vi "calibration_main.vi"() -> ()   [LabVIEW 2019]
uses:
  <vilib>/vision/Calibration.llb/Error Statistics.ctl
  LinearTransformationDescriptionCluster.ctl
  <vilib>/vision/driver/IMAQdx.llb/IMAQdx Acquisition Mode.ctl
  <vilib>/vision/Calibration.llb/Distortion Model.ctl
  <vilib>/vision/Calibration.llb/Distortion Model Types.ctl
  CalibrationStepsEnum.ctl
  CircleDetectionEnum.ctl
  <vilib>/vision/Calibration.llb/Calibration Reference Points.ctl
  radiucenter2topleftwidthheight.vi
  affine_transform_point.vi
  ParametersGlobal.vi
  <vilib>/vision/driver/NI_Vision_Acquisition_Software.lvlib
  <vilib>/vision/NI_Vision_Development_Module.lvlib
panel:
  in  "Camera":bool
  in  "Configure Projector and Calibrate Power for Tag:\n(Blank if N/A, nonblank skips Spatial Calibration)":string
  out "error out":errorcluster
  out "Parameters Written":string[][](array[string])
  in  "Power Meter Probe Area (mm^2)":dbl=71.0 format="%#_13g"
  in  "Power":bool
  out "Error Map":sgl[][](graph)
  out "distortion corrected std":dbl format="%0.2f"
  out "linear std":dbl format="%0.2f"
  out "distortion corrected error mean (camera pixels)":dbl format="%0.2f"
  out "linear mean error (camera pixels)":dbl format="%0.2f"
  out "Calibration Instructions":string="Calibration Has Not Started"
  in  "Next Step":bool
  out "Linear Tranformation Description":T1 {"mean error\n(projector pixels)" format="%0.2f"}
  out "Projector  to Camera\nError Statistics (pixels)":T2
  out "grid step (camera pixels)":dbl
  out "mean linear error\n(projector pixels)":dbl format="%0.2f"
  out "Stimulus Image":T3(plugin-control)
  out "ProjectorXY":cluster{"X":dbl, "Y":dbl}[](graph)
  out "CameraXY":cluster{"X":dbl, "Y":dbl}[](graph)
  out "CorrectionMetric":dbl
  out "Spiral Iteration":i32
  in  "ProjectedRadiusFactor":dbl=0.1 format="%#_13g"
  out "CameraToProjectorCorrection":dbl
  out "Circles Data":T4(array[cluster])
  out "Real World\nError Statistics (mm)":T5
  out "Processed Image":T3(plugin-control)
  out "Acquired Image":T3(plugin-control)
  # "Skip Calibration If Possible For:"
  # "Things you need before starting:\n(?) An agar plate with calibration grid paper with\n     0.25mm spacing (1/4 size). This is only required \n     if camera needs to be calibrated\n(?) An agar plate with plain paper\n(-) An agar plate with no paper\n(?) A power meter on an a 9cm plate (no agar)\n     This is only required for power calibration"
  # "If this % distortion is > 1%\nSomething is probably wrong"
  # "±"
  # "±"
  # "C:/Users/Public/Documents/National Instruments/Vision/Documentation/CalibrationGrid.pdf"
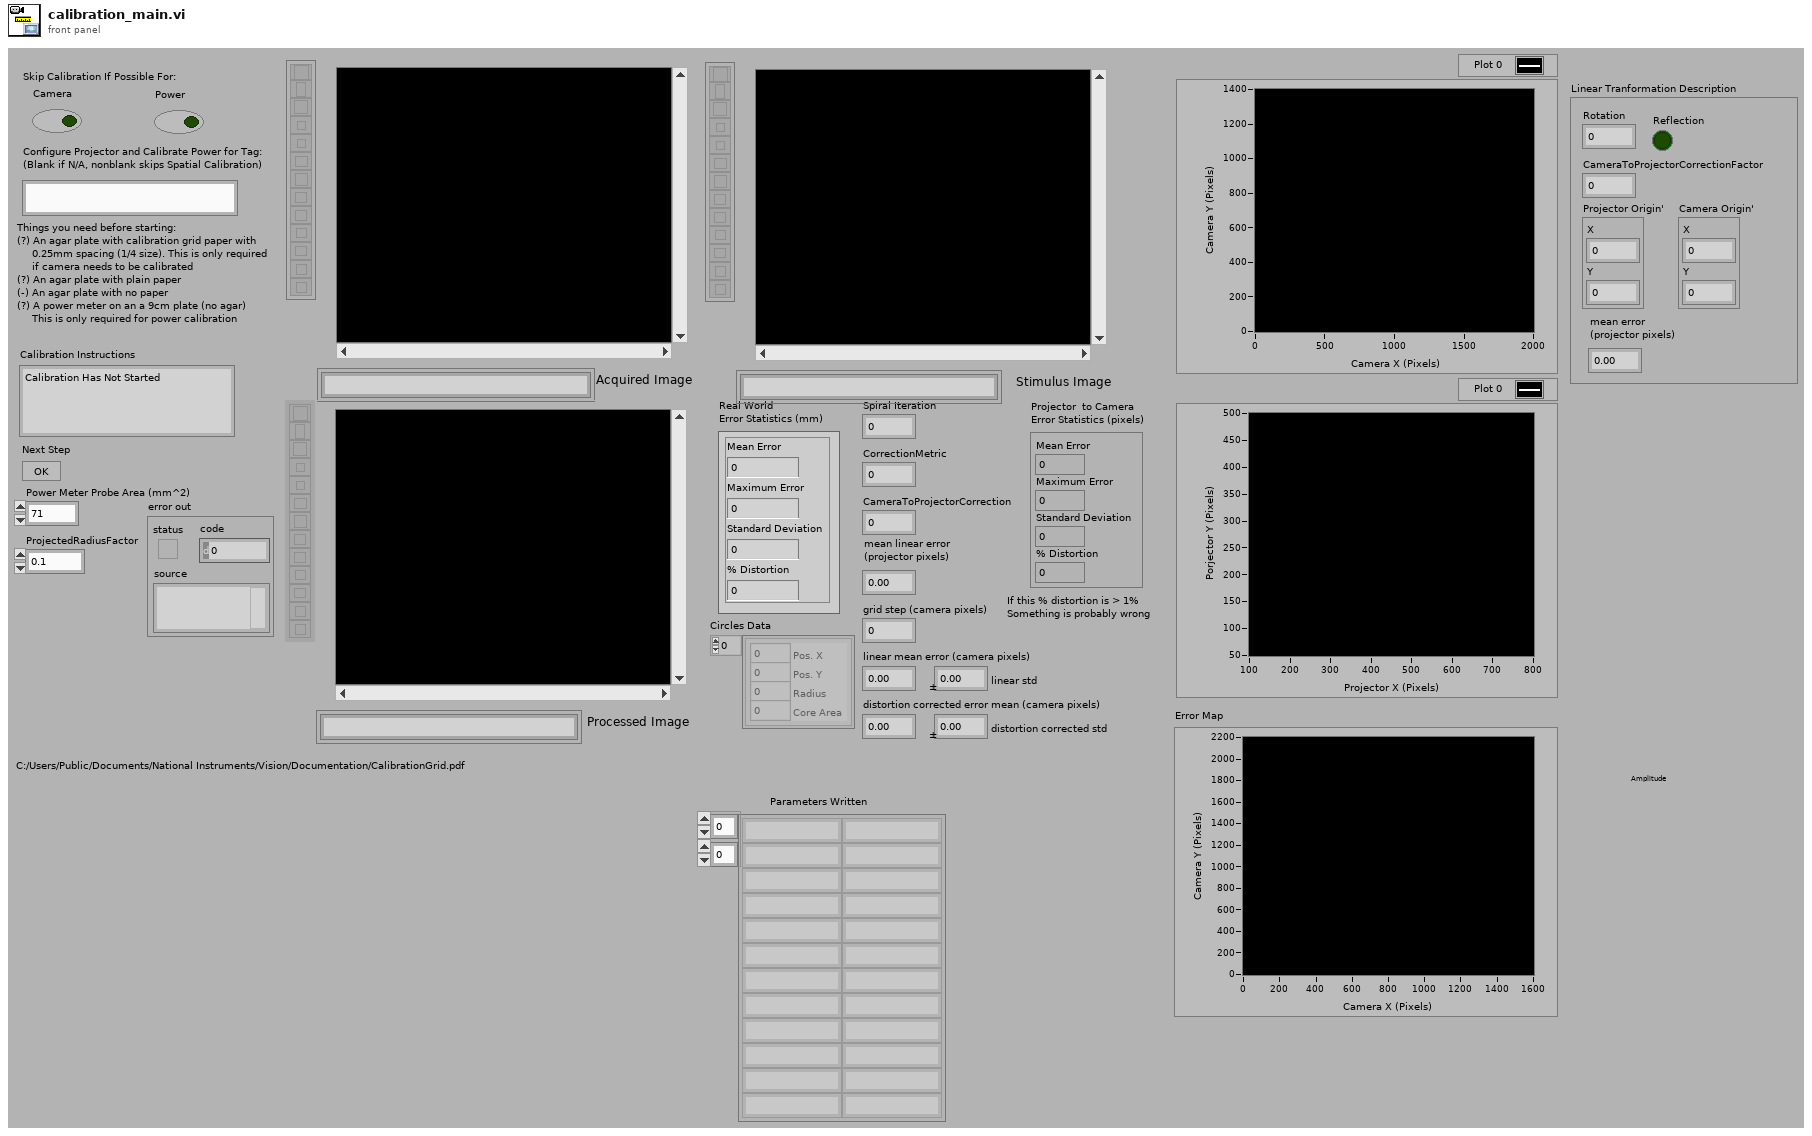
[diagram p1: front panel]
types:
  T1 = typedef "LinearTransformationDescriptionCluster.ctl" = cluster{"Rotation":sgl, "Reflection":bool, "CameraToProjectorCorrectionFactor":dbl, "Projector Origin'":cluster{"X":dbl, "Y":dbl}, "Camera Origin'":cluster{"X":dbl, "Y":dbl}, "mean error\n(projector pixels)":dbl}
  T2 = typedef "Error Statistics.ctl" = cluster{"Mean Error":dbl, "Maximum Error":dbl, "Standard Deviation":dbl, "% Distortion":dbl}
  T3 = typedef "IMAQ Image.ctl" = refnum<image>
  T4 = cluster{"Pos. X":i32, "Pos. Y":i32, "Radius":i32, "Core Area":i32}[]
  T5 = cluster{"Mean Error":dbl, "Maximum Error":dbl, "Standard Deviation":dbl, "% Distortion":dbl}
  T6 = typedef "NI_Vision_Acquisition_Software.lvlib/IMAQdx Acquisition Mode.ctl" = enum32{"One Shot", "Continuous"}
  T7 = typedef "Image Type" = u32
  T8 = typedef "IMAQdx.ctl" = refnum<k21>
  T9 = typedef "Image Unit" = enum32{"Undefined", "Angström", "Micrometer", "Millimeter", "Centimeter", "Meter", "Kilometer", "Microinch", "Inch", "Feet", "Nautical miles", "Standard miles", "Steps"}
  T10 = typedef "CalibrationStepsEnum.ctl" = enum16{"FindSpot", "SpiralScan", "CalculatingLinearTranformation", "CalculatingNonlinearTransformation", "CalibrationError", "CalibrationComplete"}
  T11 = typedef "CircleDetectionEnum.ctl" = enum16{"NoCircle", "CircleCutoff", "CircleFull"}
  T12 = enum32{"AutoM", "Close", "Dilate", "Erode", "Gradient", "Gradient in", "Gradient out", "HitMiss", "Open", "PClose", "POpen", "Thick", "Thin"}
  T13 = typedef "Calibration Reference Points.ctl" = cluster{"Pixel Coordinates":cluster{"X":dbl, "Y":dbl}[], "Real World Coordinates":cluster{"X":dbl, "Y":dbl}[], "Unit":T9, "Image Size":cluster{"X":u32, "Y":u32}}
  T14 = typedef "Distortion Model.ctl" = cluster{"Distortion Model":T15, "Polynomial Model Setup":cluster{"Radial Coefficient":u32, "Tangential Coefficients ":bool}}
  T15 = typedef "Distortion Model Types.ctl" = i32
  T16 = typedef "Particle Parameters" = i32
  T17 = cluster{"Measurement Parameter":T16, "Range Lower Value":dbl, "Range Upper Value":dbl, "Range":bool, "Measurement Type":bool}[]
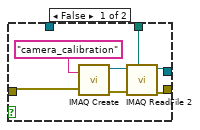
[diagram p3: hidden frame]
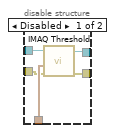
[diagram p5: hidden frame]
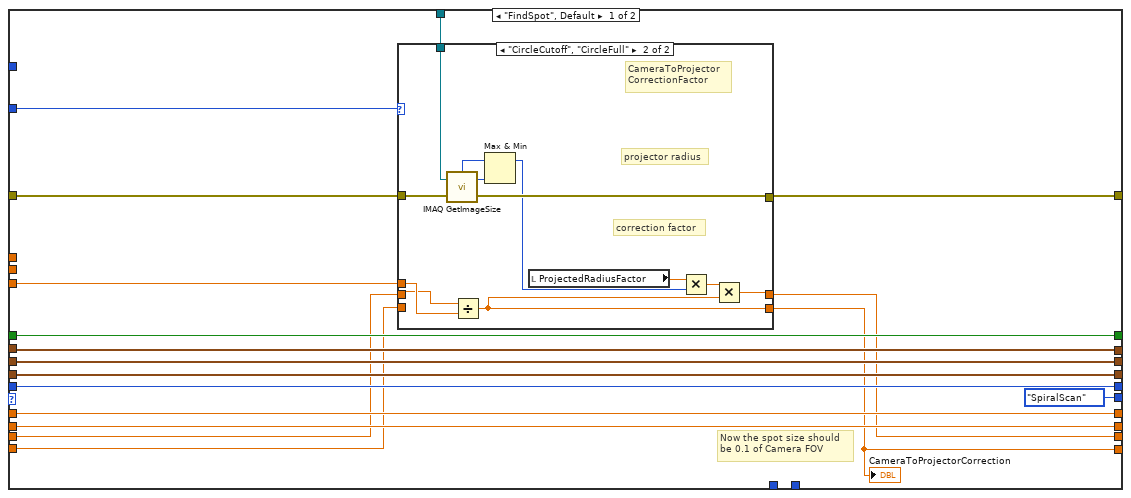
[diagram p7: hidden frame]
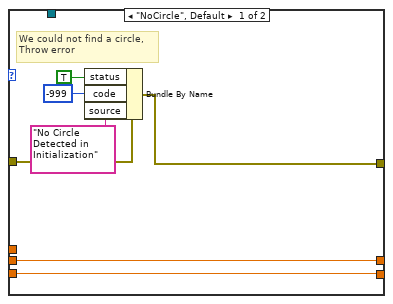
[diagram p8: hidden frame]
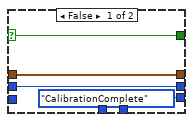
[diagram p11: hidden frame]
diagram:
  # "parameter, value pairs to update parameters.csv"
  # "computer name"
  n1 = String To IP(1:"") -> (0:w38:u32)
  n2 = IP To String(1:FALSE, 2:w38) -> (0:w37:string)
  n3 = Match Pattern(string=w37, regular expression="\\.") -> (before substring=w29:string)  [unwired: 1 in, 3 out]
  n4 = Initialize Array("", 0 ("dimension size"), 2 ("dimension size")) -> (w26:string[][])
  n5 = Not Equal?(x="Configure Projector and Calibrate Power for Tag:\n(Blank if N/A, nonblank skips Spatial Calibration)", y="") -> (x != y?=w28:bool)
  n6 = case shown="True" w28 {
    tunnel: w29 -> [w39 w43]
    tunnel: [w39 w42] -> w23
    tunnel: "Configure Projector and Calibrate Power for Tag:\n(Blank if N/A, nonblank skips Spatial Calibration)" -> [_ w45]
    frame False {
    }
    frame True {
      w41 = ";" ("delimiter")
      n7 = call <vilib>:"Space Constant.vi"() -> ("String"=w46:string)
      n8 = call <vilib>:"Delimited String to 1D String Array.vi"("delimiter"=w46, "delimited string"=w45) -> ("string array"=w44:string[])  [unwired: 9 in]
      n9 = call <vilib>:"1D String Array to Delimited String.vi"("delimiter"=w41, "string array"=w44) -> ("delimited string"=w40:string)  [unwired: 9 in]
      n10 = Concatenate Strings(w43, w41, w40) -> (w42:string)
    }
  }
  n11 = flat-sequence {
    tunnel: "Configure Projector and Calibrate Power for Tag:\n(Blank if N/A, nonblank skips Spatial Calibration)" -> [w49]
    tunnel: w26 -> [w54]
    tunnel: w23 -> [w53]
    tunnel: [w49] -> w22
    tunnel: [w54] -> w21
    tunnel: [w53] -> w20
    tunnel: [w48] -> w5
    tunnel: [w47] -> w2
    tunnel: [w110] -> w24
    tunnel: [w111] -> w25
    tunnel: w22 -> [w63]
    tunnel: w21 -> [w111]
    tunnel: w20 -> [w110]
    tunnel: [w75] -> w19
    tunnel: [w74] -> w18
    tunnel: [w66] -> w17
    tunnel: [w65] -> w16
    tunnel: [w62] -> w6
    tunnel: w2 -> [w60]
    tunnel: [w56] -> w1
    frame #0 {
      # "allow resolution mismatch"
      n12 = call "load_parameters.vi"("Create Data Folder (T)"=FALSE, "Tags"=w49) -> ("error out"=w52:errorcluster, "Computer Found"=w48:bool)  [unwired: 7 in, 1 out]
      n13 = call <vilib>:"Clear Errors.vi"("error in (no error)"=w52, "specific error code to clear (0: all)"=-919) -> ("error out"=w47:errorcluster)  [unwired: 4 in, 1 out]
      n14 = local write "Calibration Instructions"("Starting Calibration... Please Wait") -> ()
    }
    frame #1 {
      w68 = u32 20  # Number of Buffers
      w67 = IMAQdx_Acquisition_Mode."Continuous"  # Continuous?
      w81 = T7 4 items=["Grayscale (U8)", "Grayscale (I16)", "Grayscale (SGL)", "Complex (CSG)", "RGB (U32)", "HSL (U32)", "RGB (U64)"] ("Image Type")
      w77 = T7 4 items=["Grayscale (U8)", "Grayscale (I16)", "Grayscale (SGL)", "Complex (CSG)", "RGB (U32)", "HSL (U32)", "RGB (U64)"] ("Image Type")
      # "The stimulus Image has half the verticle resolution for 4500s"
      # "display full field image"
      n15 = global read "ParametersGlobal.vi" "Projector Calibration Points"() -> (w106:cluster{"X":dbl, "Y":dbl}[])
      n16 = global read "ParametersGlobal.vi" "PureGreenExposureTime"() -> (w58:i32)
      n17 = Array Size(array=w106) -> (size(s)=w107:i32)
      n18 = call "initialize_projector.vi"("Green Only"=TRUE, "error in"=w60, "green exp_time_us"=w58) -> ("error out"=w59:errorcluster)  [unwired: 8 in]
      n19 = Equal To 0?(x=w107) -> (x = 0?=w108:bool)
      n20 = Not Equal?(x=w63, y="") -> (x != y?=w62:bool)
      n21 = And(x=w108, y=w62) -> (x .and. y?=w109:bool)
      n22 = case shown="True" w109 {
        tunnel: [w115 w116] -> w64
        tunnel: w59 -> [w115 w119]
        frame False {
        }
        frame True {
          # "require tags to have previous calibration"
          n23 = call <vilib>:"Simple Error Handler.vi"("error code (no error:0)"=-723, "error source (\" \")"="Attepting to calibrate for a tag without a previous spatial calibration" ("error source (\" \")"), "error in (no error)"=w119) -> ("error out"=w116:errorcluster)  [unwired: 2 in, 4 out]
        }
      }
      n24 = call "setup_window_display.vi"("error in (no error)"=w64) -> ("error out"=w103:errorcluster, "Height"=w105:i16, "Width"=w104:i16)  [unwired: 8 in]
      n25 = case shown="Error .." w64 {
        selector: w64 -> [_ w112]
        frame No Error {
        }
        frame Error {
          n26 = flat-sequence {
            tunnel: w112 -> [w113]
            frame #0 {
              n27 = local write "error out"(w113) -> ()
            }
            frame #1 {
              n28 = Stop(stop? (T)=TRUE) -> ()
            }
          }
        }
      }
      n29 = call "IMAQ WindZoom 2"("error in (no error)"=w103, "Zoom to Fit? (False)"=TRUE ("Zoom to Fit? (T)")) -> ("error out"=w91:errorcluster)  [unwired: 6 in, 3 out]
      n30 = call "IMAQ Create"("Border Size"=0, "Image Name"="StimulusImage", "Image Type"=w81) -> ("New Image"=w92:T3, "error out"=w96:errorcluster)  [unwired: 2 in]
      n31 = call "IMAQ Create"("Border Size"=0, "Image Name"="DisplayImage", "Image Type"=w77, "error in (no error)"=w91) -> ("New Image"=w90:T3, "error out"=w89:errorcluster)  [unwired: 1 in]
      n32 = call "IMAQ SetImageSize"("error in (no error)"=w89, "Y Resolution"=w105, "X Resolution"=w104, "Image"=w90) -> ("error out"=w102:errorcluster, "Image Out"=w99:T3)  [unwired: 1 in]
      n33 = Divide(x=w105, y=2) -> (x/y=w95:dbl)
      n34 = Round Toward -Infinity(1:w95) -> (0:w94:dbl)
      n35 = global read "ParametersGlobal.vi" "IMAQdx Session"() -> (w69:T8)
      n36 = call "IMAQ SetImageSize"("error in (no error)"=w96, "Y Resolution"=w94, "X Resolution"=w104, "Image"=w92) -> ("error out"=w97:errorcluster, "Image Out"=w93:T3)  [unwired: 1 in]
      n37 = call "IMAQ FillImage"("Color Pixel Value"=u32 0, "error in (no error)"=w97, "Image"=w93) -> ("error out"=w98:errorcluster, "Image Out"=w56:T3)  [unwired: 7 in]
      n38 = local write "Next Step"(FALSE) -> ()
      n39 = call "IMAQ Expand"("Y Duplication Step"=2, "error in (no error)"=w98, "Image Dst"=w99, "Image Src"=w56) -> ("error out"=w101:errorcluster, "Image Dst Out"=w57:T3)  [unwired: 6 in]
      n40 = call <vilib>:"IMAQdx Open Camera.vi"("Session In"=w69) -> ("error out"=w72:errorcluster, "Session Out"=w73:T8)  [unwired: 9 in]
      n41 = Merge Errors(w101, w102) -> (w100:errorcluster)
      n42 = call "IMAQ WindDraw"("Resize to Image Size? (Y)"=FALSE, "error in (no error)"=w100, "Image"=w57) -> ("error out"=w75:errorcluster, "Image Out (duplicate)"=w74:T3)  [unwired: 7 in]
      n43 = call <vilib>:"IMAQdx Configure Acquisition.vi"("error in"=w72, "Number of Buffers"=w68, "Continuous?"=w67, "Session In"=w73) -> ("error out"=w71:errorcluster, "Session Out"=w70:T8)  [unwired: 6 in]
      n44 = call <vilib>:"IMAQdx Start Acquisition.vi"("error in"=w71, "Session In"=w70) -> ("error out"=w66:errorcluster, "Session Out"=w65:T8)  [unwired: 8 in]
    }
  }
  n45 = Not(x=w6) -> (.not. x?=w3:bool)
  n46 = And(x=w3, y=w5) -> (x .and. y?=w4:bool)
  n47 = case shown="True" w3 {
    tunnel: w25 -> [w126 w140]
    tunnel: w24 -> [w125 w139]
    tunnel: w1 -> [w122 w138]
    tunnel: w19 -> [w120 w137]
    tunnel: w18 -> [w121 w136]
    tunnel: w17 -> [w123 w135]
    tunnel: w16 -> [w124 w134]
    tunnel: [w125 w133] -> w13
    tunnel: [w124 w132] -> w12
    tunnel: [w122 w131] -> w11
    tunnel: [w121 w130] -> w10
    tunnel: [w120 w129] -> w9
    tunnel: [w126 w128] -> w8
    tunnel: [w123 w127] -> w7
    frame False {
    }
    frame True {
      # "do spatial calibration"
      n48 = flat-sequence {
        tunnel: [w310] -> w308
        tunnel: [w326] -> w307
        tunnel: [w325] -> w306
        tunnel: [w324] -> w305
        tunnel: [w312] -> w304
        tunnel: [w311] -> w303
        tunnel: [w323] -> w302
        tunnel: [w313] -> w301
        tunnel: [w322] -> w300
        tunnel: w134 -> [w324]
        tunnel: w135 -> [w310]
        tunnel: w136 -> [w326]
        tunnel: w137 -> [w325]
        tunnel: w138 -> [w323]
        tunnel: w140 -> [w322]
        tunnel: w139 -> [w313]
        tunnel: w308 -> [w362]
        tunnel: [w358] -> w294
        tunnel: [w383] -> w295
        tunnel: [w382] -> w296
        tunnel: w307 -> [w383]
        tunnel: w306 -> [w382]
        tunnel: w305 -> [w358]
        tunnel: w304 -> [w363]
        tunnel: w303 -> [w360]
        tunnel: [w335] -> w297
        tunnel: [w334] -> w298
        tunnel: w302 -> [w356]
        tunnel: [w356] -> w299
        tunnel: w301 -> [w343]
        tunnel: [w343] -> w293
        tunnel: w300 -> [w342]
        tunnel: [w338] -> w292
        tunnel: w299 -> [w400]
        tunnel: [w399] -> w284
        tunnel: w298 -> [w412]
        tunnel: [w412] -> w285
        tunnel: w297 -> [w411]
        tunnel: [w411] -> w286
        tunnel: w296 -> [w395]
        tunnel: [w397] -> w287
        tunnel: w295 -> [w396]
        tunnel: [w398] -> w288
        tunnel: w294 -> [w410]
        tunnel: [w410] -> w289
        tunnel: w293 -> [w408]
        tunnel: [w408] -> w290
        tunnel: w292 -> [w407]
        tunnel: [w407] -> w291
        tunnel: [w423] -> w283
        tunnel: [w422] -> w282
        tunnel: [w421] -> w281
        tunnel: [w420] -> w280
        tunnel: [w419] -> w279
        tunnel: w291 -> [w419]
        tunnel: w290 -> [w420]
        tunnel: w289 -> [w421]
        tunnel: w288 -> [w417]
        tunnel: w287 -> [w416]
        tunnel: w286 -> [w422]
        tunnel: w285 -> [w423]
        tunnel: w284 -> [w415]
        tunnel: [w417] -> w278
        tunnel: [w416] -> w277
        tunnel: [w415] -> w276
        tunnel: w283 -> [w438]
        tunnel: [w438] -> w275
        tunnel: w282 -> [w430]
        tunnel: [w428] -> w274
        tunnel: [w425] -> w273
        tunnel: [w426] -> w272
        tunnel: w281 -> [w429]
        tunnel: [w429] -> w271
        tunnel: w280 -> [w437]
        tunnel: [w437] -> w270
        tunnel: w279 -> [w436]
        tunnel: [w436] -> w269
        tunnel: [w427] -> w268
        tunnel: w278 -> [w426]
        tunnel: w277 -> [w425]
        tunnel: [w424] -> w267
        tunnel: w276 -> [w424]
        tunnel: [w440] -> w266
        tunnel: w275 -> [w456]
        tunnel: [w456] -> w265
        tunnel: w274 -> [w455]
        tunnel: [w455] -> w264
        tunnel: w273 -> [w443]
        tunnel: [w442] -> w263
        tunnel: w272 -> [w444]
        tunnel: [w441] -> w262
        tunnel: w271 -> [w454]
        tunnel: [w454] -> w261
        tunnel: w270 -> [w453]
        tunnel: [w453] -> w260
        tunnel: w269 -> [w452]
        tunnel: [w452] -> w259
        tunnel: w268 -> [w451]
        tunnel: [w451] -> w258
        tunnel: w267 -> [w439]
        tunnel: w266 -> [w473]
        tunnel: [w473] -> w257
        tunnel: w265 -> [w472]
        tunnel: [w472] -> w256
        tunnel: w264 -> [w469]
        tunnel: [w462] -> w255
        tunnel: w263 -> [w471]
        tunnel: [w471] -> w254
        tunnel: w262 -> [w470]
        tunnel: [w470] -> w253
        tunnel: w261 -> [w468]
        tunnel: [w468] -> w252
        tunnel: [w461] -> w251
        tunnel: [w460] -> w250
        tunnel: w260 -> [w460]
        tunnel: w259 -> [w459]
        tunnel: [w459] -> w249
        tunnel: [w458] -> w248
        tunnel: w258 -> [w458]
        tunnel: [w509] -> w247
        tunnel: [w508] -> w246
        tunnel: [w505] -> w245
        tunnel: w257 -> [w500]
        tunnel: w256 -> [w481]
        tunnel: w255 -> [w506]
        tunnel: w254 -> [w502]
        tunnel: w253 -> [w507]
        tunnel: w252 -> [w504]
        tunnel: [w504] -> w244
        tunnel: [w485] -> w243
        tunnel: [w484] -> w242
        tunnel: [w482] -> w241
        tunnel: [w481] -> w240
        tunnel: w251 -> [w480]
        tunnel: [w480] -> w239
        tunnel: w250 -> [w476]
        tunnel: [w476] -> w238
        tunnel: w249 -> [w475]
        tunnel: [w475] -> w237
        tunnel: w248 -> [w474]
        tunnel: w247 -> [w913]
        tunnel: [w913] -> w236
        tunnel: w246 -> [w909]
        tunnel: [w909] -> w235
        tunnel: w245 -> [w908]
        tunnel: [w907] -> w234
        tunnel: w244 -> [w912]
        tunnel: [w912] -> w233
        tunnel: w243 -> [w911]
        tunnel: w242 -> [w910]
        tunnel: [w903] -> w232
        tunnel: w241 -> [w906]
        tunnel: [w906] -> w231
        tunnel: w240 -> [w905]
        tunnel: [w905] -> w230
        tunnel: w239 -> [w904]
        tunnel: [w904] -> w229
        tunnel: [w903] -> w228
        tunnel: w238 -> [w902]
        tunnel: [w902] -> w227
        tunnel: w237 -> [w901]
        tunnel: [w901] -> w226
        tunnel: w236 -> [w960]
        tunnel: [w961] -> w225
        tunnel: w235 -> [w967]
        tunnel: [w931] -> w224
        tunnel: w234 -> [w971]
        tunnel: [w959] -> w223
        tunnel: w233 -> [w972]
        tunnel: [w972] -> w222
        tunnel: w232 -> [w956]
        tunnel: w231 -> [w968]
        tunnel: w230 -> [w958]
        tunnel: [w937] -> w221
        tunnel: [w915] -> w220
        tunnel: [w958] -> w219
        tunnel: [w916] -> w218
        tunnel: [w922] -> w217
        tunnel: w229 -> [w957]
        tunnel: [w957] -> w216
        tunnel: [w946] -> w215
        tunnel: w228 -> [w941]
        tunnel: [w941] -> w214
        tunnel: w227 -> [w933]
        tunnel: [w933] -> w213
        tunnel: w226 -> [w918]
        tunnel: [w928] -> w212
        tunnel: w225 -> [w1074]
        tunnel: [w1074] -> w211
        tunnel: w224 -> [w1073]
        tunnel: [w1073] -> w210
        tunnel: w223 -> [w1072]
        tunnel: [w1009] -> w209
        tunnel: w222 -> [w1071]
        tunnel: [w1071] -> w208
        tunnel: w221 -> [w1063]
        tunnel: w220 -> [w1062]
        tunnel: w219 -> [_]
        tunnel: w218 -> [_]
        tunnel: w217 -> [w1059]
        tunnel: w216 -> [w1067]
        tunnel: [w1067] -> w207
        tunnel: w215 -> [w992]
        tunnel: [w1052] -> w206
        tunnel: [w993] -> w205
        tunnel: w214 -> [w1065]
        tunnel: [w1065] -> w204
        tunnel: w213 -> [w1061]
        tunnel: [w1061] -> w203
        tunnel: w212 -> [w995]
        tunnel: [w1022] -> w202
        tunnel: [w1008] -> w201
        tunnel: [w1059] -> w200
        tunnel: [w1053] -> w199
        tunnel: [w1031] -> w198
        tunnel: [w992] -> w197
        tunnel: w211 -> [w1085]
        tunnel: w210 -> [w1084]
        tunnel: w209 -> [w1097]
        tunnel: [w1096] -> w186
        tunnel: w208 -> [w1102]
        tunnel: [w1102] -> w187
        tunnel: w207 -> [w1101]
        tunnel: [w1101] -> w188
        tunnel: w206 -> [w1098]
        tunnel: w205 -> [w1094]
        tunnel: w204 -> [w1099]
        tunnel: w203 -> [w1089]
        tunnel: [w1089] -> w189
        tunnel: w202 -> [w1088]
        tunnel: [w1088] -> w190
        tunnel: [w1081] -> w191
        tunnel: w201 -> [w1081]
        tunnel: w200 -> [w1086]
        tunnel: [w1086] -> w192
        tunnel: [w1085] -> w193
        tunnel: [w1084] -> w194
        tunnel: w199 -> [w1083]
        tunnel: [w1083] -> w195
        tunnel: w198 -> [w1082]
        tunnel: [w1082] -> w196
        tunnel: [w1080] -> w185
        tunnel: w197 -> [w1080]
        tunnel: [w1117] -> w184
        tunnel: [w1124] -> w183
        tunnel: [w1127] -> w182
        tunnel: [w1126] -> w181
        tunnel: [w1122] -> w180
        tunnel: [w1120] -> w179
        tunnel: [w1121] -> w178
        tunnel: [w1125] -> w177
        tunnel: [w1123] -> w176
        tunnel: [w1119] -> w175
        tunnel: [w1112] -> w174
        tunnel: [w1111] -> w173
        tunnel: w196 -> [w1119]
        tunnel: w195 -> [w1123]
        tunnel: w194 -> [w1125]
        tunnel: w193 -> [w1121]
        tunnel: w192 -> [w1120]
        tunnel: w191 -> [w1122]
        tunnel: w190 -> [w1126]
        tunnel: w189 -> [w1127]
        tunnel: w188 -> [w1124]
        tunnel: w187 -> [w1117]
        tunnel: w186 -> [w1118]
        tunnel: [w1108] -> w172
        tunnel: w185 -> [w1108]
        tunnel: [w1137] -> w171
        tunnel: [w1136] -> w170
        tunnel: w184 -> [w1149]
        tunnel: [w1149] -> w169
        tunnel: w183 -> [w1148]
        tunnel: [w1148] -> w168
        tunnel: w182 -> [w1147]
        tunnel: [w1147] -> w167
        tunnel: w181 -> [w1146]
        tunnel: [w1146] -> w166
        tunnel: w180 -> [w1145]
        tunnel: [w1145] -> w165
        tunnel: [w1138] -> w164
        tunnel: w179 -> [w1135]
        tunnel: w178 -> [w1134]
        tunnel: w177 -> [w1133]
        tunnel: w176 -> [w1132]
        tunnel: w175 -> [w1131]
        tunnel: [w1132] -> w163
        tunnel: [w1131] -> w162
        tunnel: w174 -> [w1130]
        tunnel: [w1130] -> w161
        tunnel: w173 -> [w1129]
        tunnel: [w1129] -> w160
        tunnel: [w1128] -> w159
        tunnel: w172 -> [w1128]
        tunnel: [w1173] -> w158
        tunnel: [w1185] -> w157
        tunnel: [w1160] -> w156
        tunnel: [w1184] -> w155
        tunnel: [w1180] -> w154
        tunnel: [w1178] -> w153
        tunnel: [w1170] -> w152
        tunnel: w171 -> [w1173]
        tunnel: w170 -> [w1185]
        tunnel: w169 -> [w1184]
        tunnel: w168 -> [w1174]
        tunnel: w167 -> [w1180]
        tunnel: w166 -> [w1179]
        tunnel: w165 -> [w1165]
        tunnel: w164 -> [w1170]
        tunnel: w163 -> [_]
        tunnel: w162 -> [w1171]
        tunnel: w161 -> [w1167]
        tunnel: w160 -> [w1155]
        tunnel: w159 -> [w1154]
        tunnel: [w1154] -> w151
        tunnel: [w1153] -> w150
        tunnel: w158 -> [w1197]
        tunnel: [w1197] -> w141
        tunnel: w157 -> [w1196]
        tunnel: [w1196] -> w142
        tunnel: w156 -> [w1195]
        tunnel: [w1195] -> w143
        tunnel: w155 -> [w1194]
        tunnel: [w1194] -> w144
        tunnel: w154 -> [w1193]
        tunnel: [w1193] -> w145
        tunnel: w153 -> [w1192]
        tunnel: [w1192] -> w146
        tunnel: w152 -> [w1191]
        tunnel: [w1191] -> w147
        tunnel: w151 -> [w1190]
        tunnel: [w1190] -> w148
        tunnel: w150 -> [w1189]
        tunnel: [w1189] -> w149
        tunnel: [w1212] -> w133
        tunnel: [w1211] -> w132
        tunnel: [w1206] -> w131
        tunnel: [w1207] -> w130
        tunnel: [w1208] -> w129
        tunnel: [w1210] -> w128
        tunnel: [w1209] -> w127
        tunnel: w149 -> [w1204]
        tunnel: w148 -> [w1205]
        tunnel: w147 -> [w1206]
        tunnel: w146 -> [w1210]
        tunnel: w145 -> [w1212]
        tunnel: w144 -> [w1211]
        tunnel: w143 -> [w1203]
        tunnel: w142 -> [w1208]
        tunnel: w141 -> [w1207]
        frame #0 {
          n49 = Concatenate Strings("..\\", w313, "_camera_calibration.png") -> (w316:string)
          n50 = Current VI's Path() -> (path=w320:path)
          n51 = Build Path(base path=w320, name or relative path=w316) -> (appended path=w311:path)
          n52 = call <vilib>:"Check if File or Folder Exists.vi"("path"=w311) -> ("file or folder exists?"=w319:bool)  [unwired: 8 in, 2 out]
          n53 = Not(x="Camera") -> (.not. x?=w314:bool)
          n54 = Not(x=w319) -> (.not. x?=w318:bool)
          n55 = Or(x=w318, y=w314) -> (x .or. y?=w312:bool)
          n56 = local write "Calibration Instructions"("Load dot calibration plate. Turn on IR") -> ()
          n57 = while {
            tunnel: w312 -> [w328]
            stop <- w330 stop-if-true
            n58 = local read "Next Step"() -> (w329:bool)
            n59 = Not(x=w328) -> (.not. x?=w327:bool)
            n60 = Wait (ms)(milliseconds to wait=500) -> ()  [unwired: 1 out]
            n61 = Or(x=w327, y=w329) -> (x .or. y?=w330:bool)
          }
        }
        frame #1 {
          w373 = T14 {"Distortion Model"=0, "Polynomial Model Setup"={"Radial Coefficient"=1, "Tangential Coefficients "=TRUE}}  # Distortion Model Setup
          w374 = T17 [{"Measurement Parameter"=35, "Range Lower Value"=0.0, "Range Upper Value"=1000.0, "Range"=FALSE, "Measurement Type"=FALSE}, {"Measurement Parameter"=49, "Range Lower Value"=0.0, "Range Upper Value"=95.0, "Range"=FALSE, "Measurement Type"=FALSE}]  # Particle Filter Selection Values
          w376 = TRUE  # Remove Particles
          w375 = TRUE  # Reject Border?
          w380 = u32 1 items=["Bright Objects", "Dark Objects"] ("Look For (Bright Objects)")
          # "Calibrate the camera with real world 2.5mm spacing dots"
          n62 = case shown="True" w363 {
            tunnel: w362 -> [w389 w394]
            tunnel: [w386 w393] -> w361
            tunnel: [w387 w392] -> w359
            tunnel: w360 -> [w384 _]
            tunnel: w358 -> [_ w391]
            frame False {
              n63 = call "IMAQ Create"("Image Name"="camera_calibration", "error in (no error)"=w389) -> ("New Image"=w385:T3, "error out"=w388:errorcluster)  [unwired: 2 in, 1 out]
              n64 = call "IMAQ ReadFile 2"("File Path"=w384, "error in (no error)"=w388, "Image"=w385) -> ("error out"=w387:errorcluster, "Image Out"=w386:T3)  [unwired: 4 in, 3 out]
            }
            frame True {
              n65 = call "snap_single_image.vi"("error in (no error)"=w394, "Session In"=w391) -> ("error out"=w392:errorcluster, "Image Out"=w393:T3)  [unwired: 8 in]
            }
          }
          n66 = call-poly "IMAQ Write File 2"("error in (no error)"=w359, "File Path"=w360, "Image"=w361) -> ("error out"=w352:errorcluster, "Image Out (duplicate)"=w337:T3)  [unwired: 7 in]
          n67 = local write "Acquired Image"(w337) -> ()
          n68 = call "IMAQ Create"("Image Name"="cameacalibration", "error in (no error)"=w352) -> ("New Image"=w354:T3, "error out"=w351:errorcluster)  [unwired: 3 in]
          n69 = call "IMAQ Local Threshold"("Image Src"=w337, "Look For (Bright Objects)"=w380, "Image Dst"=w354, "Window Size (32x32)"=cluster{"SizeX":i32, "SizeY":i32} {"SizeX"=100, "SizeY"=100}, "error in (no error)"=w351) -> ("Image Dst Out"=w364:T3, "error out"=w372:errorcluster)  [unwired: 4 in, 5 out]
          n70 = call "IMAQ Particle Filter 3"("Image Src"=w364, "Selection Values"=w374, "Keep/Remove Particles (F)"=w376, "error in (no error)"=w372, "Reject Border? (F)"=w375) -> ("Image Dst Out"=w365:T3, "error out"=w371:errorcluster)  [unwired: 4 in, 5 out]
          n71 = call "IMAQ Calibration Target to Points - Circular Dots 2"("error in (no error)"=w371, "Grid Descriptor"=cluster{"X Step":sgl, "Y Step":sgl, "Unit":T9} {"X Step"=2.5, "Y Step"=2.5, "Unit"=enum."Millimeter"}, "Target Image"=w365) -> ("error out"=w370:errorcluster, "Reference Points"=w353:T13, "Target Image (dup)"=w379:T3)  [unwired: 6 in]
          n72 = call "IMAQ Learn Distortion Model"("Distortion Model Setup"=w373, "error in (no error)"=w370, "Reference Points"=w353, "Calibration Template Image"=w379) -> ("error out"=w369:errorcluster, "Calibration Template Image Out"=w378:T3)  [unwired: 2 in, 4 out]
          n73 = call "IMAQ Learn Perspective Calibration"("error in (no error)"=w369, "Reference Points"=w353, "Calibration Template Image"=w378) -> ("error out"=w366:errorcluster, "Calibration Template Image Out"=w368:T3)  [unwired: 1 in, 6 out]
          n74 = Concatenate Strings("..\\", w343, "_camera_distortion.png") -> (w341:string)
          n75 = local write "Next Step"(FALSE) -> ()
          n76 = Current VI's Path() -> (path=w347:path)
          n77 = call "IMAQ Get Calibration Info 3"("Calibration Template Image"=w368, "Return Error Information (False)"=TRUE, "error in (no error)"=w366) -> ("Calibration Template Image (duplicate)"=w348:T3, "Error Statistics"=→"Real World\nError Statistics (mm)":T2, "error out"=w349:errorcluster)  [unwired: 4 in, 6 out]
          n78 = Build Path(base path=w347, name or relative path=w341) -> (appended path=w346:path)
          n79 = Build Array("CameraCalibrationImagePath" ("element"), w341) -> (w339:string[])
          n80 = call "IMAQ Write Image And Vision Info File 2"("error in (no error)"=w349, "File Path"=w346, "Image"=w348) -> ("error out"=w336:errorcluster, "Image Out (duplicate)"=w334:T3)  [unwired: 7 in]
          n81 = Build Array (concatenate)(w342, w339) -> (w338:string[][])
          n82 = call "IMAQ UserLookup 2"("Image Src"=w334, "Lookup Table"=i32[] [0, 255], "error in (no error)"=w336) -> ("Image Dst Out"=w332:T3, "error out"=w335:errorcluster)  [unwired: 4 in]
          n83 = local write "Processed Image"(w332) -> ()
        }
        frame #2 {
          n84 = while {
            stop <- w413 stop-if-true
            n85 = local read "Next Step"() -> (w413:bool)
            n86 = Wait (ms)(milliseconds to wait=500) -> ()  [unwired: 1 out]
          }
          n87 = call "IMAQ FillImage"("Color Pixel Value"=u32 65280, "error in (no error)"=w395, "Image"=w400) -> ("error out"=w402:errorcluster, "Image Out"=w399:T3)  [unwired: 7 in]
          n88 = local write "Calibration Instructions"("Load paper on agar plate. Turn off IR.\nIf this step fails repeatedly, try tuning\nthe ProjectedRadiusFactor. ") -> ()
          n89 = call "IMAQ Expand"("Y Duplication Step"=2, "error in (no error)"=w402, "Image Dst"=w396, "Image Src"=w399) -> ("error out"=w404:errorcluster, "Image Dst Out"=w403:T3)  [unwired: 6 in]
          n90 = call "IMAQ WindDraw"("Resize to Image Size? (Y)"=FALSE, "error in (no error)"=w404, "Image"=w403) -> ("error out"=w397:errorcluster, "Image Out (duplicate)"=w398:T3)  [unwired: 7 in]
        }
        frame #3 {
          # "get full field green image"
          n91 = local write "Next Step"(FALSE) -> ()
        }
        frame #4 {
          n92 = call "snap_single_image.vi"("error in (no error)"=w430, "Session In"=w429) -> ("error out"=w434:errorcluster, "Image Out"=w431:T3)  [unwired: 8 in]
          n93 = call "IMAQ Create"("Image Name"="fullgreen", "error in (no error)"=w434) -> ("New Image"=w433:T3, "error out"=w432:errorcluster)  [unwired: 3 in]
          n94 = call "IMAQ Copy"("error in (no error)"=w432, "Image Dst"=w433, "Image Src"=w431) -> ("error out"=w428:errorcluster, "Image Dst Out"=w427:T3)  [unwired: 3 in]
          n95 = local write "Acquired Image"(w427) -> ()
        }
        frame #5 {
          n96 = call "IMAQ FillImage"("Color Pixel Value"=u32 0, "error in (no error)"=w443, "Image"=w439) -> ("error out"=w446:errorcluster, "Image Out"=w440:T3)  [unwired: 7 in]
          n97 = flat-sequence {
            tunnel: w442 -> [_]
            frame #0 {
              # "display update delay"
              n98 = Wait (ms)(milliseconds to wait=1500) -> ()  [unwired: 1 out]
            }
          }
          n99 = call "IMAQ Expand"("Y Duplication Step"=2, "error in (no error)"=w446, "Image Dst"=w444, "Image Src"=w440) -> ("error out"=w448:errorcluster, "Image Dst Out"=w447:T3)  [unwired: 6 in]
          n100 = call "IMAQ WindDraw"("Resize to Image Size? (Y)"=FALSE, "error in (no error)"=w448, "Image"=w447) -> ("error out"=w442:errorcluster, "Image Out (duplicate)"=w441:T3)  [unwired: 7 in]
        }
        frame #6 {
          # "get background image"
          n101 = call "snap_single_image.vi"("error in (no error)"=w469, "Session In"=w468) -> ("error out"=w466:errorcluster, "Image Out"=w463:T3)  [unwired: 8 in]
          n102 = call "IMAQ Create"("Image Name"="background", "error in (no error)"=w466) -> ("New Image"=w465:T3, "error out"=w464:errorcluster)  [unwired: 3 in]
          n103 = call "IMAQ Copy"("error in (no error)"=w464, "Image Dst"=w465, "Image Src"=w463) -> ("error out"=w462:errorcluster, "Image Dst Out"=w461:T3)  [unwired: 3 in]
          n104 = local write "Acquired Image"(w461) -> ()
        }
        frame #7 {
          w488 = 0
          # "empty point arrays"
          # "Current Calibration Step"
          # "Should we go to the next spiral iteration?\nthat is, a full circle was found in the last iteration"
          # "CameraToProjectorCorrectionFactor"
          # "spiral iteration #"
          # "y center"
          # "x center"
          # "radius"
          # "Initialize as center of projector\nwith a radius of 0.1 times the\nlarger stimulus dimension, \nassuming the\ncorrection factor is 1"
          n105 = call "IMAQ GetImageSize"("Image"=w500, "error in (no error)"=w502) -> ("Y Resolution"=w490:i32, "X Resolution"=w491:i32, "error out"=w501:errorcluster)  [unwired: 2 in]
          n106 = Max & Min(x=w491, y=w490) -> (max(x,y)=w503:i32)  [unwired: 1 out]
          n107 = Divide(x=w491, y=2) -> (x/y=w499:dbl)
          n108 = Divide(x=w490, y=2) -> (x/y=w497:dbl)
          n109 = Round Toward -Infinity(1:w499) -> (0:w495:dbl)
          n110 = Round Toward -Infinity(1:w497) -> (0:w494:dbl)
          n111 = Multiply(x=w503, y="ProjectedRadiusFactor") -> (x*y=w493:dbl)
          n112 = call "SquareSpiral.vi"("Height"=w490, "Width"=w491, "Iteration Number"=w488, "SpiralThickness (0 to 1)"="ProjectedRadiusFactor") -> ("ProjectorCoordinates"=w487:cluster{"X":dbl, "Y":dbl}[])
          n113 = Initialize Array(cluster{"X":dbl, "Y":dbl} {"X"=0.0, "Y"=0.0}, 0) -> (w478:cluster{"X":dbl, "Y":dbl}[])
          n114 = while {
            shift-right: [w594] -> w509
            shift-left: w507 -> [w591]
            shift-right: [w593] -> w508
            shift-left: w501 -> [w590]
            shift-right: [w511] -> w505
            shift-left: w506 -> [w589]
            tunnel: w504 -> [w588]
            shift-right: [w580] -> _
            shift-left: w495 -> [w584]
            shift-right: [w578] -> _
            shift-left: w494 -> [w583]
            shift-right: [w576] -> _
            shift-left: w493 -> [w582]
            shift-right: [w546] -> _
            shift-left: CalibrationStepsEnum."FindSpot" -> [w560]
            shift-right: [w552] -> w482
            shift-left: w500 -> [w592]
            shift-right: [w551] -> _
            shift-left: 1.0 -> [w550]
            shift-right: [w538] -> _
            shift-left: w488 -> [w542]
            shift-right: [w521] -> _
            shift-left: w487 -> [w536]
            shift-right: [w520] -> w484
            shift-left: w478 -> [w533]
            shift-right: [w519] -> w485
            shift-left: w478 -> [w531]
            shift-right: [w518] -> _
            shift-left: FALSE -> [w529]
            tunnel: w480 -> [w514]
            tunnel: w480 -> [w512]
            tunnel: w474 -> [w510]
            stop <- w543 stop-if-true
            n115 = flat-sequence {
              tunnel: w592 -> [w622]
              tunnel: w591 -> [w618]
              tunnel: w590 -> [w617]
              tunnel: [w631] -> w575
              tunnel: [w630] -> w573
              tunnel: w589 -> [w615]
              tunnel: [w615] -> w571
              tunnel: [w599] -> w569
              tunnel: w584 -> [w612]
              tunnel: w583 -> [w613]
              tunnel: w582 -> [w614]
              tunnel: [w612] -> w567
              tunnel: [w613] -> w565
              tunnel: [w614] -> w563
              tunnel: [w611] -> w561
              tunnel: w560 -> [w611]
              tunnel: w550 -> [w606]
              tunnel: [w606] -> w549
              tunnel: w542 -> [w605]
              tunnel: [w605] -> w541
              tunnel: [w604] -> w537
              tunnel: w536 -> [w604]
              tunnel: [w603] -> w534
              tunnel: w533 -> [w603]
              tunnel: [w602] -> w532
              tunnel: w531 -> [w602]
              tunnel: [w601] -> w530
              tunnel: w529 -> [w601]
              tunnel: w575 -> [w646]
              tunnel: [w646] -> w574
              tunnel: w573 -> [w645]
              tunnel: [w645] -> w572
              tunnel: w571 -> [w644]
              tunnel: [w644] -> w570
              tunnel: w569 -> [w643]
              tunnel: [w643] -> w568
              tunnel: w567 -> [w642]
              tunnel: [w642] -> w566
              tunnel: w565 -> [w641]
              tunnel: [w641] -> w564
              tunnel: w563 -> [w640]
              tunnel: [w640] -> w562
              tunnel: w561 -> [w638]
              tunnel: [w638] -> w559
              tunnel: w549 -> [w637]
              tunnel: [w637] -> w548
              tunnel: w541 -> [w636]
              tunnel: [w636] -> w540
              tunnel: w537 -> [w635]
              tunnel: [w635] -> w535
              tunnel: w534 -> [w634]
              tunnel: w532 -> [w633]
              tunnel: w530 -> [w632]
              tunnel: [w634] -> w528
              tunnel: [w633] -> w527
              tunnel: [w632] -> w526
              tunnel: w574 -> [w710]
              tunnel: w572 -> [w707]
              tunnel: w570 -> [w709]
              tunnel: w588 -> [w708]
              tunnel: w568 -> [w679]
              tunnel: [w710] -> w587
              tunnel: [w707] -> w586
              tunnel: [w659] -> w585
              tunnel: w566 -> [w701]
              tunnel: w564 -> [w700]
              tunnel: w562 -> [w699]
              tunnel: [w701] -> w581
              tunnel: [w700] -> w579
              tunnel: [w699] -> w577
              tunnel: w559 -> [w691]
              tunnel: [w691] -> w558
              tunnel: [w687] -> w557
              tunnel: [w686] -> w556
              tunnel: [w685] -> w555
              tunnel: [w680] -> w554
              tunnel: [w679] -> w553
              tunnel: w548 -> [w678]
              tunnel: [w678] -> w547
              tunnel: w540 -> [w677]
              tunnel: [w677] -> w539
              tunnel: w535 -> [w673]
              tunnel: w528 -> [w674]
              tunnel: w527 -> [w675]
              tunnel: w526 -> [w676]
              tunnel: [w676] -> w525
              tunnel: [w675] -> w524
              tunnel: [w674] -> w523
              tunnel: [w673] -> w522
              tunnel: [w665] -> w517
              tunnel: w514 -> [w666]
              tunnel: w510 -> [w650]
              tunnel: [w764] -> w511
              tunnel: [w742] -> w593
              tunnel: [w771] -> w594
              tunnel: w587 -> [w771]
              tunnel: w586 -> [w743]
              tunnel: w585 -> [w765]
              tunnel: w581 -> [w769]
              tunnel: [w763] -> w580
              tunnel: w579 -> [w768]
              tunnel: [w762] -> w578
              tunnel: w577 -> [w767]
              tunnel: [w761] -> w576
              tunnel: w558 -> [w770]
              tunnel: w557 -> [w746]
              tunnel: w556 -> [w745]
              tunnel: w555 -> [w759]
              tunnel: w554 -> [w766]
              tunnel: [w760] -> w546
              tunnel: w553 -> [w744]
              tunnel: [w744] -> w552
              tunnel: [w758] -> w551
              tunnel: w547 -> [w757]
              tunnel: w539 -> [w755]
              tunnel: [w756] -> w538
              tunnel: w525 -> [w751]
              tunnel: w524 -> [w752]
              tunnel: w523 -> [w753]
              tunnel: w522 -> [w754]
              tunnel: [w750] -> w521
              tunnel: [w749] -> w520
              tunnel: [w748] -> w519
              tunnel: [w747] -> w518
              tunnel: w517 -> [w739]
              tunnel: w512 -> [w738]
              frame #0 {
                w629 = u16 1 items=["Frame", "Paint", "Invert Frame", "Invert Paint"] ("Draw Mode")
                w628 = u16 2 items=["Line", "Rectangle", "Oval"] ("Shape to draw")
                # "display update delay"
                # "draw pause"
                # "green"
                # "CameraXY with Full Circles"
                # "ProjectorXY With Full Circles"
                # "ProjectorXY To Try"
                # "draw the circle on the projector"
                n116 = call "IMAQ FillImage"("Color Pixel Value"=u32 0, "error in (no error)"=w617, "Image"=w622) -> ("error out"=w620:errorcluster, "Image Out"=w621:T3)  [unwired: 7 in]
                n117 = call "radiucenter2boundingbox.vi"("Radius"=w614, "ycenter"=w613, "xcenter"=w612) -> ("Bottom"=w607:i32, "Right"=w608:i32, "Top"=w609:i32, "Left"=w610:i32)  [unwired: 2 in]
                n118 = Build Array(w610, w609, w608, w607) -> (w626:i32[])
                n119 = call "IMAQ Draw"("Draw Mode"=w629, "Shape to draw"=w628, "Pixel Color"=65280, "error in (no error)"=w620, "Coordinates"=w626, "Image Src"=w621) -> ("error out"=w619:errorcluster, "Image Dst Out"=w599:T3)  [unwired: 4 in]
                n120 = local write "Stimulus Image"(w599) -> ()
                n121 = call "IMAQ Expand"("Y Duplication Step"=2, "error in (no error)"=w619, "Image Dst"=w618, "Image Src"=w599) -> ("error out"=w616:errorcluster, "Image Dst Out"=w624:T3)  [unwired: 6 in]
                n122 = Wait (ms)(milliseconds to wait=150) -> ()  [unwired: 1 out]
                n123 = call "IMAQ WindDraw"("Resize to Image Size? (Y)"=FALSE, "error in (no error)"=w616, "Image"=w624) -> ("error out"=w630:errorcluster, "Image Out (duplicate)"=w631:T3)  [unwired: 7 in]
              }
              frame #1 {
                # "Display\nPause"
                n124 = Wait (ms)(milliseconds to wait=200) -> ()  [unwired: 1 out]
              }
              frame #2 {
                # "Keep the biggest circle"
                # "The smallest circle is a half of the PRF"
                # "extract the circle from the camera"
                n125 = global read "ParametersGlobal.vi" "CalibrationBinaryThresholdLevel (out of 255)"() -> (w654:dbl)
                n126 = call "snap_single_image.vi"("error in (no error)"=w709, "Session In"=w708) -> ("error out"=w669:errorcluster, "Image Out"=w667:T3)  [unwired: 8 in]
                n127 = call "IMAQ Create"("Image Name"="processed", "error in (no error)"=w669) -> ("New Image"=w652:T3, "error out"=w668:errorcluster)  [unwired: 3 in]
                n128 = call "IMAQ Subtract"("Image Src A"=w667, "Image Dst"=w652, "Image Src B"=w666, "error in (no error)"=w668) -> ("Image Dst Out"=w649:T3, "error out"=w651:errorcluster)  [unwired: 3 in]
                n129 = Bundle By Name(cluster=cluster{"Lower value":sgl, "Upper value":sgl} {"Lower value"=100.0, "Upper value"=255.0} ("Range"), "Lower value"=w654) -> (w655:cluster{"Lower value":sgl, "Upper value":sgl})
                n130 = call "IMAQ MulDiv"("Image Src A"=w649, "Image Dst"=w649, "Image Src B"=w650, "error in (no error)"=w651) -> ("Image Dst Out"=w647:T3, "error out"=w648:errorcluster)  [unwired: 3 in]
                n131 = disable-structure shown="Enabled" {
                  disable-tunnel: [w715 w719] -> w662
                  disable-tunnel: [w714 w720] -> w661
                  disable-tunnel: w655 -> [w713 w716]
                  disable-tunnel: w648 -> [w712 w717]
                  disable-tunnel: w647 -> [w711 w718]
                  frame Disabled {
                    n132 = call "IMAQ Threshold"("error in (no error)"=w712, "Range"=w713, "Image Src"=w711) -> ("error out"=w714:errorcluster, "Image Dst Out"=w715:T3)  [unwired: 7 in]
                  }
                  frame Enabled {
                    n133 = call "IMAQ AutoBThreshold 2"("Image Src"=w718, "error in (no error)"=w717, "Threshold Limits"=w716) -> ("Image Dst Out"=w719:T3, "error out"=w720:errorcluster)  [unwired: 10 in, 1 out]
                  }
                }
                n134 = local read "ProjectedRadiusFactor"() -> (w672:dbl)
                n135 = call "IMAQ FillHole"("error in (no error)"=w661, "Image Src"=w662) -> ("error out"=w663:errorcluster, "Image Dst Out"=w664:T3)  [unwired: 4 in]
                n136 = local write "Acquired Image"(w667) -> ()
                n137 = call "IMAQ GetImageSize"("Image"=w664, "error in (no error)"=w663) -> ("Y Resolution"=w705:i32, "X Resolution"=w704:i32, "error out"=w706:errorcluster)  [unwired: 2 in]
                n138 = Max & Min(x=w704, y=w705) -> (max(x,y)=w665:i32)  [unwired: 1 out]
                n139 = Divide(x=w672, y=2.0) -> (x/y=w670:dbl)
                n140 = Multiply(x=w665, y=w670) -> (x*y=w703:dbl)
                n141 = call "IMAQ Find Circles"("Max Radius"=w665, "error in (no error)"=w706, "Min Radius"=w703, "Image Src"=w664) -> ("error out"=w697:errorcluster, "Circles Data"=w695:T4, "Nb Circles"=w690:i32, "Image Dst Out"=w698:T3)  [unwired: 4 in]
                "Circles Data" <- w695
                n142 = call "IMAQ GrayMorphology"("error in (no error)"=w697, "Operation"=T12."Dilate", "Image Src"=w698) -> ("error out"=w660:errorcluster, "Image Dst Out"=w653:T3)  [unwired: 7 in]
                n143 = for {
                  tunnel: w695 -> [w731] mode=indexing
                  shift-right: [w726] -> w687
                  shift-left: 0.0 -> [w728]
                  shift-right: [w725] -> w686
                  shift-left: 0.0 -> [w729]
                  shift-right: [w724] -> w685
                  shift-left: 0.0 -> [w727]
                  n144 = Unbundle By Name(w731) -> ("Pos. X"=w723:i32, "Pos. Y"=w722:i32, "Radius"=w721:i32)
                  n145 = Greater Or Equal?(x=w721, y=w727) -> (x >= y?=w730:bool)
                  n146 = case shown="True" w730 {
                    tunnel: w729 -> [w733 _]
                    tunnel: w728 -> [w734 _]
                    tunnel: w727 -> [w732 _]
                    tunnel: [w734 w735] -> w726
                    tunnel: [w733 w736] -> w725
                    tunnel: [w732 w737] -> w724
                    tunnel: w723 -> [_ w735]
                    tunnel: w722 -> [_ w736]
                    tunnel: w721 -> [_ w737]
                    frame False {
                    }
                    frame True {
                    }
                  }
                }
                n147 = local write "Processed Image"(w653) -> ()
                n148 = call "IMAQ GetImageSize"("Image"=w653, "error in (no error)"=w660) -> ("Y Resolution"=w658:i32, "X Resolution"=w657:i32, "error out"=w659:errorcluster)  [unwired: 2 in]
                n149 = call "radiucenterinbound.vi"("Y Resolution"=w658, "xcenter"=w687, "ycenter"=w686, "Radius"=w685, "X Resolution"=w657) -> ("WithinBounds"=w684:bool)  [unwired: 3 in]
                n150 = Equal To 0?(x=w690) -> (x = 0?=w689:bool)
                n151 = Select(t=CircleDetectionEnum."CircleFull", s=w684, f=CircleDetectionEnum."CircleCutoff") -> (s? t:f=w681:T11)
                n152 = Select(t=CircleDetectionEnum."NoCircle", s=w689, f=w681) -> (s? t:f=w680:T11)
              }
              frame #3 {
                n153 = call "IMAQ GetImageSize"("Image"=w744, "error in (no error)"=w743) -> ("Y Resolution"=w740:i32, "X Resolution"=w741:i32, "error out"=w742:errorcluster)  [unwired: 2 in]
                n154 = case shown="\"SpiralScan\"" w770 {
                  selector: w770 -> [_ w840]
                  tunnel: w769 -> [w783 w830]
                  tunnel: w768 -> [w782 w829]
                  tunnel: w767 -> [w776 w828]
                  tunnel: w766 -> [w788 w813]
                  tunnel: w765 -> [w787 w811]
                  tunnel: [w786 w811] -> w764
                  tunnel: [w783 w832] -> w763
                  tunnel: [w782 w831] -> w762
                  tunnel: [w775 w828] -> w761
                  tunnel: [CalibrationStepsEnum."SpiralScan" w833] -> w760
                  tunnel: w759 -> [w784 w820]
                  tunnel: [w774 w827] -> w758
                  tunnel: w757 -> [w773 w827]
                  tunnel: [w781 w826] -> w756
                  tunnel: w755 -> [w781 w839]
                  tunnel: w754 -> [w780 w843]
                  tunnel: w753 -> [w779 w848]
                  tunnel: w752 -> [w778 w845]
                  tunnel: w751 -> [w777 w842]
                  tunnel: [w780 w834] -> w750
                  tunnel: [w779 w824] -> w749
                  tunnel: [w778 w825] -> w748
                  tunnel: [w777 w836] -> w747
                  tunnel: w746 -> [_ w847]
                  tunnel: w745 -> [_ w846]
                  tunnel: w741 -> [_ w838]
                  tunnel: w740 -> [_ w837]
                  tunnel: w739 -> [_ w823]
                  tunnel: w738 -> [w772 _]
                  frame "FindSpot", Default {
                    # "Now the spot size should\nbe 0.1 of Camera FOV"
                    n155 = case shown="\"CircleCutoff\", \"CircleFull\"" w788 {
                      tunnel: w787 -> [w794 w803]
                      tunnel: [w795 w802] -> w786
                      tunnel: w784 -> [_ w807]
                      tunnel: w776 -> [w790 w806]
                      tunnel: [w790 w805] -> w775
                      tunnel: [w789 w804] -> w774
                      tunnel: w773 -> [w789 _]
                      tunnel: w772 -> [_ w801]
                      frame "NoCircle", Default {
                        # "We could not find a circle,\nThrow error"
                        n156 = Bundle By Name(cluster=w794, "status"=TRUE, "code"=-999, "source"="No Circle Detected in Initialization") -> (w795:errorcluster)
                      }
                      frame "CircleCutoff", "CircleFull" {
                        # "correction factor"
                        # "projector radius"
                        # "CameraToProjector\nCorrectionFactor"
                        n157 = call "IMAQ GetImageSize"("Image"=w801, "error in (no error)"=w803) -> ("Y Resolution"=w800:i32, "X Resolution"=w799:i32, "error out"=w802:errorcluster)  [unwired: 2 in]
                        n158 = Divide(x=w806, y=w807) -> (x/y=w804:dbl)
                        n159 = Max & Min(x=w799, y=w800) -> (max(x,y)=w797:i32)  [unwired: 1 out]
                        n160 = local read "ProjectedRadiusFactor"() -> (w796:dbl)
                        n161 = Multiply(x=w796, y=w797) -> (x*y=w798:dbl)
                        n162 = Multiply(x=w798, y=w804) -> (x*y=w805:dbl)
                      }
                    }
                    "CameraToProjectorCorrection" <- w774
                  }
                  frame "SpiralScan" {
                    # "Check to see if our crude\nCameraToProjectorCorrectionFactor\nis off by a lot. If not, then add the point"
                    n163 = local read "ProjectedRadiusFactor"() -> (w822:dbl)
                    n164 = Multiply(x=w823, y=w822) -> (x*y=w821:dbl)
                    n165 = Divide(x=w821, y=w820) -> (x/y=w819:dbl)
                    "CorrectionMetric" <- w819
                    n166 = Less?(x=w819, y=0.7) -> (x < y?=w815:bool)
                    n167 = Greater?(x=w819, y=1.3) -> (0:w816:bool)
                    n168 = Equal?(x=w813, y=CircleDetectionEnum."CircleFull") -> (x = y?=w814:bool)
                    n169 = Or(x=w816, y=w815) -> (x .or. y?=w808:bool)
                    n170 = Not(x=w808) -> (.not. x?=w809:bool)
                    n171 = And(x=w809, y=w814) -> (x .and. y?=w810:bool)
                    n172 = case shown="True" w810 {
                      tunnel: w848 -> [w886 w898]
                      tunnel: w830 -> [_ w897]
                      tunnel: w829 -> [_ w896]
                      tunnel: w847 -> [_ w893]
                      tunnel: w846 -> [_ w892]
                      tunnel: w845 -> [w887 w890]
                      tunnel: w842 -> [w888 _]
                      tunnel: [w888 TRUE] -> w841
                      tunnel: [w887 w891] -> w825
                      tunnel: [w886 w899] -> w824
                      frame False {
                      }
                      frame True {
                        w894 = cluster{"X":dbl, "Y":dbl} {"X"=0.0, "Y"=0.0}
                        # "Record the XY positions of circles\nin POV and FOV, one more spiral"
                        n173 = Bundle By Name(cluster=w894, "X"=w897, "Y"=w896) -> (w895:cluster{"X":dbl, "Y":dbl})
                        n174 = Bundle By Name(cluster=w894, "X"=w893, "Y"=w892) -> (w889:cluster{"X":dbl, "Y":dbl})
                        n175 = Build Array (concatenate)(w898, w895) -> (w899:cluster{"X":dbl, "Y":dbl}[])
                        n176 = Build Array (concatenate)(w890, w889) -> (w891:cluster{"X":dbl, "Y":dbl}[])
                      }
                    }
                    n177 = Empty Array?(array=w843) -> (empty?=w844:bool)
                    n178 = case shown="True" w844 {
                      tunnel: w843 -> [w860 w864]
                      tunnel: w841 -> [w861 w873]
                      tunnel: [w863 w872] -> w833
                      tunnel: w840 -> [w863 w871]
                      tunnel: w839 -> [w862 w870]
                      tunnel: [w862 w869] -> w826
                      tunnel: [w860 w868] -> w835
                      tunnel: w838 -> [_ w867]
                      tunnel: w837 -> [_ w866]
                      tunnel: [w861 w865] -> w836
                      frame False {
                        # "We are not done with this spiral\niteration yet, keep going"
                      }
                      frame True {
                        # "Spiral Iteration Complete"
                        n179 = case shown="True" w873 {
                          selector: w873 -> [w875 _]
                          tunnel: [CalibrationStepsEnum."CalibrationComplete" w885] -> w872
                          tunnel: w871 -> [_ w885]
                          tunnel: w870 -> [w876 w884]
                          tunnel: [w876 w882] -> w869
                          tunnel: [w874 w883] -> w868
                          tunnel: w867 -> [_ w881]
                          tunnel: w866 -> [_ w880]
                          tunnel: [w875 FALSE] -> w865
                          tunnel: w864 -> [w874 _]
                          frame False {
                          }
                          frame True {
                            # "We found a full circle\nin this iteration"
                            n180 = local read "ProjectedRadiusFactor"() -> (w879:dbl)
                            n181 = Increment(x=w884) -> (x+1=w882:i32)
                            n182 = call "SquareSpiral.vi"("Height"=w880, "Width"=w881, "Iteration Number"=w882, "SpiralThickness (0 to 1)"=w879) -> ("ProjectorCoordinates"=w883:cluster{"X":dbl, "Y":dbl}[])
                          }
                        }
                      }
                    }
                    n183 = case shown="\"SpiralScan\", Default" w833 {
                      tunnel: w835 -> [w852 w859]
                      tunnel: [w853 w859] -> w834
                      tunnel: [w850 w858] -> w832
                      tunnel: [w849 w857] -> w831
                      tunnel: w830 -> [_ w858]
                      tunnel: w829 -> [_ w857]
                      frame "SpiralScan", Default {
                        # "Load the next element\nof the spiral"
                        n184 = Index Array(array=w852, index=0) -> (element=w851:cluster{"X":dbl, "Y":dbl})
                        n185 = Unbundle By Name(w851) -> ("X"=w850:dbl, "Y"=w849:dbl)
                        n186 = Delete From Array(array=w852, length=1, index=0) -> (array with subset deleted=w853:cluster{"X":dbl, "Y":dbl}[])  [unwired: 1 out]
                      }
                      frame "CalibrationComplete" {
                        # "We are done, no more\nelements left"
                      }
                    }
                  }
                }
              }
            }
            n187 = Unbundle By Name(w511) -> ("source"=w515:string, "status"=w516:bool)
            n188 = case shown="Error .." w511 {
              selector: w511 -> [_ w595]
              frame No Error {
              }
              frame Error {
                n189 = flat-sequence {
                  tunnel: w595 -> [w596]
                  frame #0 {
                    n190 = local write "error out"(w596) -> ()
                  }
                  frame #1 {
                    n191 = Stop(stop? (T)=TRUE) -> ()
                  }
                }
              }
            }
            n192 = local write "Calibration Instructions"(w515) -> ()
            n193 = Wait (ms)(milliseconds to wait=0) -> ()  [unwired: 1 out]
            n194 = Equal?(x=CalibrationStepsEnum."CalibrationComplete", y=w546) -> (x = y?=w544:bool)
            n195 = Or(x=w516, y=w544) -> (x .or. y?=w543:bool)
            "Spiral Iteration" <- w538
          }
        }
        frame #8 {
          # "Calculate linear\ntranformation from\nstimulus space to \ncamera space"
          n196 = call "ProjectorCameraXY2LinearTransformation.vi"("error in (no error)"=w908, "ProjectorXY"=w910, "CameraXY"=w911) -> ("error out"=w907:errorcluster, "Linear Tranformation Description"=w903:T1)  [unwired: 6 in]
          "CameraXY" <- w911
          "ProjectorXY" <- w910
        }
        frame #9 {
          # "Y"
          # "X"
          # "delta"
          # "Border size (Camera pixels)"
          # "CameraXY"
          # "Draw a dot grid with the projector"
          # "draw on projector"
          # "Build Grid with border inside camera's FOV"
          # "dot radius"
          # "X Grid Count"
          n197 = call "IMAQ GetImageSize"("Image"=w958, "error in (no error)"=w971) -> ("Y Resolution"=w947:i32, "X Resolution"=w943:i32, "error out"=w959:errorcluster)  [unwired: 2 in]
          n198 = Unbundle By Name(w956) -> ("CameraToProjectorCorrectionFactor"=w966:dbl, "mean error\n(projector pixels)"=→"mean linear error\n(projector pixels)":dbl)
          n199 = call "IMAQ FillImage"("Color Pixel Value"=u32 0, "error in (no error)"=w967, "Image"=w968) -> ("error out"=w952:errorcluster, "Image Out"=w923:T3)  [unwired: 7 in]
          n200 = Add(x=25.0, y=2.0) -> (x+y=w942:dbl)
          n201 = Divide(x=w943, y=w942) -> (x/y=w916:dbl)
          "grid step (camera pixels)" <- w916
          n202 = Divide(x=w916, y=8.0) -> (x/y=w946:dbl)
          n203 = Subtract(x=w947, y=w916) -> (x-y=w948:dbl)
          n204 = Number To Fractional String(number=w916) -> (F-format string=w921:string)  [unwired: 3 in]
          n205 = Subtract(x=w943, y=w916) -> (x-y=w949:dbl)
          n206 = call "ramp_by_delta_double.vi"("start"=w916, "end"=w949, "delta"=w916) -> ("Ramp Pattern"=w950:dbl[])  [unwired: 8 in]
          n207 = call "ramp_by_delta_double.vi"("start"=w916, "end"=w948, "delta"=w916) -> ("Ramp Pattern"=w970:dbl[])  [unwired: 8 in]
          n208 = Multiply(x=w946, y=w966) -> (x*y=w926:dbl)
          n209 = Initialize Array(cluster{"X":dbl, "Y":dbl} {"X"=0.0, "Y"=0.0}, 0) -> (w938:cluster{"X":dbl, "Y":dbl}[])
          n210 = for {
            tunnel: w970 -> [w984]
            tunnel: w950 -> [w985] mode=indexing
            shift-right: [w982] -> w937
            shift-left: w938 -> [w983]
            # "X"
            n211 = for {
              tunnel: w985 -> [w991]
              tunnel: w984 -> [w990] mode=indexing
              shift-right: [w988] -> w982
              shift-left: w983 -> [w989]
              # "Y"
              n212 = Bundle By Name(cluster=cluster{"X":dbl, "Y":dbl} {"X"=0.0, "Y"=0.0}, "X"=w991, "Y"=w990) -> (w987:cluster{"X":dbl, "Y":dbl})
              n213 = Build Array (concatenate)(w989, w987) -> (w988:cluster{"X":dbl, "Y":dbl}[])
            }
          }
          n214 = Concatenate Strings("..\\", w933, "_linear_transformation.xml") -> (w934:string)
          n215 = Flatten To XML(anything=w956) -> (xml string=w951:string)
          n216 = Current VI's Path() -> (path=w954:path)
          n217 = Build Array("SpatialCalibrationCameraStepSize" ("element"), w921) -> (w920:string[])
          n218 = Build Path(base path=w954, name or relative path=w934) -> (appended path=w953:path)
          n219 = disable-structure shown="Disabled" {
            disable-tunnel: w953 -> [w979 _]
            disable-tunnel: w952 -> [w978 w980]
            disable-tunnel: [w977 w980] -> w925
            disable-tunnel: w951 -> [w976 _]
            frame Disabled {
              n220 = Write to Text File(file (use dialog)=w979, text=w976, error in=w978) -> (error out=w977:errorcluster)  [unwired: 1 in, 2 out]
            }
            frame Enabled {
            }
          }
          n221 = Build Array (concatenate)(w918, w920) -> (w917:string[][])
          n222 = To Long Integer(number=w926) -> (32bit integer=w914:i32)
          n223 = for {
            tunnel: [w975] -> w915 mode=indexing
            tunnel: w956 -> [w974]
            tunnel: w937 -> [w973] mode=indexing
            n224 = call "CameraXY2projectorXY.vi"("Linear Transformation Description"=w974, "Camera Point"=w973) -> ("Projector Point"=w975:cluster{"X":sgl, "Y":sgl})  [unwired: 9 in]
          }
          n225 = global write "ParametersGlobal.vi" "Calibration Projector Dot Radius (projector pixel)"(w914) -> ()
          n226 = Number To Fractional String(number=w914) -> (F-format string=w927:string)  [unwired: 3 in]
          n227 = local write "ProjectorXY"(w915) -> ()
          n228 = global write "ParametersGlobal.vi" "Projector Calibration Points"(w915) -> ()
          n229 = call "generate_spatial_calibration_pattern.vi"("error in (no error)"=w925, "Dot Radius (Projector Pixels)"=w914, "Points Array"=w915, "StimulusImageIn"=w923) -> ("error out"=w924:errorcluster, "StimulusImageOut"=w922:T3)  [unwired: 6 in]
          n230 = Build Array("SpatialCalibrationProjectorDotRadius" ("element"), w927) -> (w929:string[])
          n231 = flat-sequence {
            tunnel: w931 -> [_]
            frame #0 {
              # "display update delay"
              n232 = Wait (ms)(milliseconds to wait=200) -> ()  [unwired: 1 out]
            }
          }
          n233 = local write "Stimulus Image"(w922) -> ()
          n234 = call "IMAQ Expand"("Y Duplication Step"=2, "error in (no error)"=w924, "Image Dst"=w960, "Image Src"=w922) -> ("error out"=w962:errorcluster, "Image Dst Out"=w964:T3)  [unwired: 6 in]
          n235 = Build Array (concatenate)(w917, w929) -> (w928:string[][])
          n236 = call "IMAQ WindDraw"("Resize to Image Size? (Y)"=FALSE, "error in (no error)"=w962, "Image"=w964) -> ("error out"=w931:errorcluster, "Image Out (duplicate)"=w961:T3)  [unwired: 7 in]
          "Linear Tranformation Description" <- w956
        }
        frame #10 {
          w1003 = T7 0 items=["Grayscale (U8)", "Grayscale (I16)", "Grayscale (SGL)", "Complex (CSG)", "RGB (U32)", "HSL (U32)", "RGB (U64)", "Grayscale (U16)"] ("Image Type")
          w1006 = 1 items=["Red", "Green", "Blue", "Hue", "Saturation", "Luminance", "Value", "Intensity"] ("Color Plane")
          w1010 = u16 0 items=["RGB", "HSL", "HSV", "HSI"] ("Color Mode")
          w1019 = T7 4 items=["Grayscale (U8)", "Grayscale (I16)", "Grayscale (SGL)", "Complex (CSG)", "RGB (U32)", "HSL (U32)", "RGB (U64)", "Grayscale (U16)"] ("Image Type")
          w1028 = u16 0 items=["RGB", "HSL", "HSV", "HSI"] ("Color Mode")
          w1039 = T7 4 items=["Grayscale (U8)", "Grayscale (I16)", "Grayscale (SGL)", "Complex (CSG)", "RGB (U32)", "HSL (U32)", "RGB (U64)", "Grayscale (U16)"] ("Image Type")
          w1070 = T14 {"Distortion Model"=0, "Polynomial Model Setup"={"Radial Coefficient"=1, "Tangential Coefficients "=TRUE}}  # Distortion Model Setup
          # "sort it!"
          # "extract the dot matrix information and use it as a calibration\nProjector Pixel Coordinates is \"Real World\"\nCamera Pixel Coordinates is \"Pixel Coordinates\""
          n237 = call "snap_single_image.vi"("error in (no error)"=w1072, "Session In"=w1071) -> ("error out"=w1043:errorcluster, "Image Out"=w1066:T3)  [unwired: 8 in]
          n238 = local write "Acquired Image"(w1066) -> ()
          n239 = call "IMAQ Create"("Image Name"="papercalibration", "error in (no error)"=w1043) -> ("New Image"=w1041:T3, "error out"=w1042:errorcluster)  [unwired: 3 in]
          n240 = call "IMAQ Subtract"("Image Src A"=w1066, "Image Dst"=w1041, "Image Src B"=w1067, "error in (no error)"=w1042) -> ("Image Dst Out"=w1031:T3, "error out"=w1034:errorcluster)  [unwired: 3 in]
          n241 = call "extract_calibration_standard_point_locations.vi"("error in (no error)"=w1034, "expected dot radius (camera pixels)"=w992, "Image Src"=w1031) -> ("error out"=w1035:errorcluster, "Particle Measurements (Pixels)"=w1044:dbl[][], "Image Out (duplicate)"=w1023:T3)  [unwired: 6 in]
          n242 = for {
            tunnel: w1044 -> [w1078] mode=indexing
            tunnel: [w1075] -> w1045 mode=indexing
            n243 = Index Array(array=w1078) -> (element #1=w1077:dbl, element #2=w1076:dbl)  [unwired: 2 in]
            n244 = Bundle(cluster=cluster{"X":dbl, "Y":dbl} {"X"=0.0, "Y"=0.0}, "X"=w1077, "Y"=w1076) -> (w1075:cluster{"X":dbl, "Y":dbl})
          }
          n245 = call "IMAQ Create"("Image Name"="projectorcalibration", "Image Type"=w1039, "error in (no error)"=w1035) -> ("New Image"=w1037:T3, "error out"=w1038:errorcluster)  [unwired: 2 in]
          n246 = call "IMAQ GetImageSize"("Image"=w1023, "error in (no error)"=w1038) -> ("Y Resolution"=w1032:i32, "X Resolution"=w1033:i32, "error out"=w1036:errorcluster)  [unwired: 2 in]
          n247 = call "sort_points_iterative_closest_point.vi"("Detected Camera Coordinates"=w1045, "Anticipated Camera Coordinates"=w1063, "Corresponding Projector Coordinates"=w1062) -> ("Detected Camera Coordinates Sorted"=w993:cluster{"X":dbl, "Y":dbl}[], "Corresponding Projector Coordinates Filtered"=w1052:cluster{"X":dbl, "Y":dbl}[])
          n248 = call "IMAQ SetImageSize"("error in (no error)"=w1036, "Y Resolution"=w1032, "X Resolution"=w1033, "Image"=w1037) -> ("error out"=w1030:errorcluster, "Image Out"=w1029:T3)  [unwired: 1 in]
          n249 = Bundle By Name(cluster=T13 {"Pixel Coordinates"=[], "Real World Coordinates"=[], "Unit"=enum."Undefined", "Image Size"={"X"=0, "Y"=0}} ("Reference Points"), "Real World Coordinates"=w1052, "Pixel Coordinates"=w993, "Image Size.X"=w1033, "Image Size.Y"=w1032) -> (w1046:T13)
          n250 = call "IMAQ Learn Perspective Calibration"("error in (no error)"=w1030, "Reference Points"=w1046, "Calibration Template Image"=w1029) -> ("error out"=w1056:errorcluster, "Calibration Template Image Out"=w1057:T3)  [unwired: 1 in, 6 out]
          n251 = call "points_to_semicolon_delimited_string.vi"("Array"=w993) -> ("delimited string"=w997:string)  [unwired: 10 in]
          n252 = call "IMAQ Learn Distortion Model"("Distortion Model Setup"=w1070, "error in (no error)"=w1056, "Reference Points"=w1046, "Calibration Template Image"=w1057) -> ("error out"=w1055:errorcluster, "Calibration Template Image Out"=w1054:T3)  [unwired: 2 in, 4 out]
          n253 = Build Array("CameraSpatialCalibrationPoints" ("element"), w997) -> (w998:string[])
          n254 = Build Array (concatenate)(w995, w998) -> (w994:string[][])
          n255 = local write "CameraXY"(w993) -> ()
          n256 = call "IMAQ Get Calibration Info 3"("Calibration Template Image"=w1054, "Return Error Information (False)"=TRUE, "error in (no error)"=w1055) -> ("Error Map"=→"Error Map":sgl[][], "Calibration Template Image (duplicate)"=w1008:T3, "Error Statistics"=→"Projector  to Camera\nError Statistics (pixels)":T2, "error out"=w1021:errorcluster)  [unwired: 4 in, 5 out]
          n257 = call "calibration_image_to_conversion_ratio.vi"("error in (no error)"=w1021, "Calibration Image"=w1008) -> ("error out"=w1013:errorcluster, "conversion ratio"=w1060:dbl)  [unwired: 8 in]
          n258 = Round Toward +Infinity(x=w1060) -> ()  [unwired: 1 out]
          n259 = call "points_to_semicolon_delimited_string.vi"("Array"=w1052) -> ("delimited string"=w1050:string)  [unwired: 10 in]
          n260 = local write "ProjectorXY"(w1052) -> ()
          n261 = To Long Integer(number=w1060) -> (32bit integer=w1053:i32)
          n262 = Build Array("ProjectorSpatialCalibrationPoints" ("element"), w1050) -> (w1051:string[])
          n263 = call "IMAQ Create"("Image Name"="processed_two", "Image Type"=w1019, "error in (no error)"=w1013) -> ("New Image"=w1015:T3, "error out"=w1014:errorcluster)  [unwired: 2 in]
          n264 = Build Array (concatenate)(w994, w1051) -> (w1022:string[][])
          n265 = call "IMAQ GetImageSize"("Image"=w1008, "error in (no error)"=w1014) -> ("Y Resolution"=w1017:i32, "X Resolution"=w1016:i32, "error out"=w1018:errorcluster)  [unwired: 2 in]
          n266 = call "IMAQ SetImageSize"("error in (no error)"=w1018, "Y Resolution"=w1017, "X Resolution"=w1016, "Image"=w1015) -> ("error out"=w1011:errorcluster, "Image Out"=w1012:T3)  [unwired: 1 in]
          n267 = call "projector_image_to_camera_image_subvi.vi"("Camera dot radius"=w1053, "error in (no error)"=w1011, "Converted Camera Image In"=w1012, "Projector Image In"=w1059, "Projector to Camera Calibration"=w1008) -> ("error out"=w1027:errorcluster, "Converted Camera Image Out"=w1026:T3)  [unwired: 5 in]
          n268 = call "IMAQ ReplaceColorPlane"("Image Src"=w1026, "Color Mode"=w1028, "Red or Hue Plane"=w1023, "error in (no error)"=w1027) -> ("Image Dst Out"=w1024:T3, "error out"=w1025:errorcluster)  [unwired: 10 in]
          n269 = call "IMAQ ColorEqualize"("error in (no error)"=w1025, "Luma / RGB,HSL (Luma)"=TRUE, "Image Src"=w1024) -> ("error out"=w1001:errorcluster, "Image Dst Out"=w999:T3)  [unwired: 2 in]
          n270 = call "IMAQ Create"("Image Name"="processed_green", "Image Type"=w1003, "error in (no error)"=w1001) -> ("New Image"=w1002:T3, "error out"=w1000:errorcluster)  [unwired: 2 in]
          n271 = local write "Processed Image"(w999) -> ()
          n272 = call "IMAQ ExtractSingleColorPlane"("Color Plane"=w1006, "error in (no error)"=w1000, "Image Dst"=w1002, "Image Src"=w999) -> ("error out"=w1007:errorcluster, "Image Dst Out"=w1005:T3)  [unwired: 6 in]
          n273 = call "IMAQ ReplaceColorPlane"("Image Src"=w1008, "Color Mode"=w1010, "Green or Sat Plane"=w1005, "error in (no error)"=w1007) -> ("error out"=w1009:errorcluster)  [unwired: 10 in, 1 out]
        }
        frame #11 {
          # "image of paper spatial calibration"
          # "camera dot radius"
          # "projector to camera calibration"
          # "camera session"
          # "background image"
          # "computer + tag"
          # "compare error of linear and nonlinear calibrations"
          n274 = for {
            tunnel: w1098 -> [w1107] mode=indexing
            tunnel: [w1106] -> w1100 mode=indexing
            tunnel: w1099 -> [w1105]
            n275 = call "projectorXY2CameraXY.vi"("Linear Transformation Description Template"=w1105, "Projector Point"=w1107) -> ("Camera Point"=w1106:cluster{"X":sgl, "Y":sgl})  [unwired: 9 in]
          }
          n276 = while {
            stop <- w1103 stop-if-true
            n277 = local read "Next Step"() -> (w1103:bool)
            n278 = Wait (ms)(milliseconds to wait=u32 500) -> ()  [unwired: 1 out]
          }
          n279 = call "IMAQ Convert Real World to Pixel"("error in (no error)"=w1097, "Array of Real World Coordinates"=w1098, "Calibrated Image"=w1081) -> ("error out"=w1096:errorcluster, "Array of Pixel Coordinates"=w1095:cluster{"X":sgl, "Y":sgl}[])  [unwired: 3 in, 4 out]
          n280 = call "mean_point_distance.vi"("Pointset 1"=w1095, "Pointset 2"=w1094) -> ("standard deviation"=→"distortion corrected std":dbl, "mean distance"=→"distortion corrected error mean (camera pixels)":dbl)
          n281 = call "mean_point_distance.vi"("Pointset 1"=w1094, "Pointset 2"=w1100) -> ("standard deviation"=→"linear std":dbl, "mean distance"=→"linear mean error (camera pixels)":dbl)
          n282 = local write "Calibration Instructions"("Confirm proper red/green overlap. If recalibration is required, stop VI and rerun.\n Load Plain Agar Plate. Turn on IR.") -> ()
        }
        frame #12 {
          # "display spatial calibration\npattern on agar"
          n283 = call "snap_single_image.vi"("error in (no error)"=w1118, "Session In"=w1117) -> ("error out"=w1114:errorcluster, "Image Out"=w1110:T3)  [unwired: 8 in]
          n284 = local write "Acquired Image"(w1110) -> ()
          n285 = local write "Next Step"(FALSE ("Next Step")) -> ()
          n286 = call "IMAQ Create"("Image Name"="processedagar", "error in (no error)"=w1114) -> ("New Image"=w1113:T3, "error out"=w1115:errorcluster)  [unwired: 3 in]
          n287 = call "IMAQ Copy"("error in (no error)"=w1115, "Image Dst"=w1113, "Image Src"=w1110) -> ("error out"=w1112:errorcluster, "Image Dst Out"=w1111:T3)  [unwired: 3 in]
        }
        frame #13 {
          n288 = call "IMAQ FillImage"("Color Pixel Value"=u32 0, "error in (no error)"=w1133, "Image"=w1135) -> ("error out"=w1140:errorcluster, "Image Out"=w1138:T3)  [unwired: 7 in]
          n289 = flat-sequence {
            tunnel: w1136 -> [_]
            frame #0 {
              n290 = Wait (ms)(milliseconds to wait=u32 200) -> ()  [unwired: 1 out]
            }
          }
          n291 = call "IMAQ Expand"("Y Duplication Step"=2, "error in (no error)"=w1140, "Image Dst"=w1134, "Image Src"=w1138) -> ("error out"=w1142:errorcluster, "Image Dst Out"=w1141:T3)  [unwired: 6 in]
          n292 = call "IMAQ WindDraw"("Resize to Image Size? (Y)"=FALSE, "error in (no error)"=w1142, "Image"=w1141) -> ("error out"=w1136:errorcluster, "Image Out (duplicate)"=w1137:T3)  [unwired: 7 in]
        }
        frame #14 {
          w1172 = u16 0 items=["RGB", "HSL", "HSV", "HSI"] ("Color Mode")
          # "get background of plain agar"
          # "plain agar is blue, paper is red, projector image is green"
          # "display and save calibration standard"
          n293 = call "snap_single_image.vi"("error in (no error)"=w1167, "Session In"=w1184) -> ("error out"=w1169:errorcluster, "Image Out"=w1152:T3)  [unwired: 8 in]
          n294 = call "IMAQ Copy"("error in (no error)"=w1169, "Image Dst"=w1174, "Image Src"=w1152) -> ("error out"=w1168:errorcluster, "Image Dst Out"=w1156:T3)  [unwired: 3 in]
          n295 = local write "Acquired Image"(w1152) -> ()
          n296 = call "IMAQ Subtract"("Image Src A"=w1155, "Image Dst"=w1155, "Image Src B"=w1156, "error in (no error)"=w1168) -> ("Image Dst Out"=w1153:T3, "error out"=w1166:errorcluster)  [unwired: 3 in]
          n297 = disable-structure shown="Disabled" {
            frame Disabled {
              # "detect xy shift and change the blue if needed"
              n298 = call "IMAQ Shift"() -> ()  [unwired: 10 in, 2 out]
            }
            frame Enabled {
            }
          }
          n299 = local write "Calibration Instructions"("Confirm proper red/green/blue overlap. If recalibration is required, stop VI and rerun.") -> ()
          n300 = Concatenate Strings("..\\", w1180, "_projector_to_camera_distortion.png") -> (w1175:string)
          n301 = call "IMAQ ReplaceColorPlane"("Image Src"=w1165, "Color Mode"=w1172, "Red or Hue Plane"=w1171, "error in (no error)"=w1166, "Blue or Luma or Val or Inten Plane"=w1153) -> ("Image Dst Out"=w1151:T3, "error out"=w1164:errorcluster)  [unwired: 9 in]
          n302 = Current VI's Path() -> (path=w1176:path)
          n303 = Build Array("ProjectorCameraCalibrationImagePath" ("element"), w1175) -> (w1181:string[])
          n304 = Build Path(base path=w1176, name or relative path=w1175) -> (appended path=w1163:path)
          n305 = while {
            stop <- w1186 stop-if-true
            n306 = local read "Next Step"() -> (w1186:bool)
            n307 = Wait (ms)(milliseconds to wait=u32 500) -> ()  [unwired: 1 out]
          }
          n308 = global write "ParametersGlobal.vi" "Projector Camera Calibration Image"(w1151) -> ()
          n309 = call "IMAQ Write Image And Vision Info File 2"("error in (no error)"=w1164, "File Path"=w1163, "Image"=w1151) -> ("error out"=w1161:errorcluster, "Image Out (duplicate)"=w1159:T3)  [unwired: 7 in]
          n310 = Build Array (concatenate)(w1179, w1181) -> (w1178:string[][])
          n311 = call "IMAQ ColorEqualize"("error in (no error)"=w1161, "Luma / RGB,HSL (Luma)"=TRUE, "Image Src"=w1159) -> ("error out"=w1160:errorcluster, "Image Dst Out"=w1158:T3)  [unwired: 2 in]
          n312 = local write "Processed Image"(w1158) -> ()
        }
        frame #15 {
          n313 = local write "Next Step"(FALSE ("Next Step")) -> ()
        }
        frame #16 {
          n314 = call "extract_calibration_standard_point_locations.vi"("error in (no error)"=w1203, "expected dot radius (camera pixels)"=w1205, "Image Src"=w1204) -> ("error out"=w1202:errorcluster, "Image Out (duplicate)"=w1201:T3)  [unwired: 6 in, 1 out]
          n315 = while {
            stop <- w1213 stop-if-true
            n316 = local read "Next Step"() -> (w1213:bool)
            n317 = Wait (ms)(milliseconds to wait=u32 500) -> ()  [unwired: 1 out]
          }
          n318 = call "IMAQ UserLookup 2"("Image Src"=w1201, "Lookup Table"=i32[] [0, 255], "error in (no error)"=w1202) -> ("Image Dst Out"=w1199:T3, "error out"=w1209:errorcluster)  [unwired: 4 in]
          n319 = local write "Calibration Instructions"("Confirm good binary threshold for agar. If recalibration is required, stop VI and rerun.") -> ()
          n320 = local write "Processed Image"(w1199) -> ()
        }
      }
    }
  }
  n321 = flat-sequence {
    tunnel: [w1235] -> w15
    tunnel: [w1228] -> w14
    tunnel: w8 -> [w1221]
    tunnel: w13 -> [w1237]
    tunnel: w12 -> [w1225]
    tunnel: w11 -> [w1224]
    tunnel: w10 -> [w1223]
    tunnel: w9 -> [w1222]
    tunnel: w7 -> [w1219]
    tunnel: w4 -> [w1216]
    frame #0 {
      # "power calibration"
      n322 = And(x="Power", y=w1216) -> (x .and. y?=w1217:bool)
      n323 = case shown="False" w1217 {
        tunnel: [w1313 w1578] -> w1233
        tunnel: [w1310 w1580] -> w1232
        tunnel: w1222 -> [w1332 w1580]
        tunnel: w1223 -> [w1334 _]
        tunnel: w1224 -> [w1333 _]
        tunnel: [w1295 _] -> w1227
        tunnel: [w1294 _] -> w1226
        tunnel: [w1309 _] -> w1229
        tunnel: w1225 -> [w1308 w1579]
        tunnel: [w1297 w1579] -> w1234
        tunnel: w1219 -> [w1275 w1578]
        tunnel: [w1258 _] -> w1215
        frame False {
          n324 = flat-sequence {
            tunnel: w1275 -> [w1336]
            tunnel: w1334 -> [w1337]
            tunnel: w1333 -> [w1338]
            tunnel: w1332 -> [w1339]
            tunnel: w1308 -> [w1340]
            tunnel: [w1340] -> w1263
            tunnel: [w1339] -> w1262
            tunnel: [w1338] -> w1261
            tunnel: [w1337] -> w1260
            tunnel: [w1336] -> w1259
            tunnel: [w1363] -> w1273
            tunnel: [w1349] -> w1271
            tunnel: [w1346] -> w1269
            tunnel: [w1348] -> w1267
            tunnel: [w1355] -> w1265
            tunnel: w1263 -> [w1363]
            tunnel: w1262 -> [w1350]
            tunnel: w1261 -> [w1347]
            tunnel: w1260 -> [w1351]
            tunnel: w1259 -> [w1356]
            tunnel: [w1343] -> w1258
            tunnel: [w1368] -> w1274
            tunnel: w1273 -> [w1369]
            tunnel: [w1369] -> w1272
            tunnel: w1271 -> [w1378]
            tunnel: [w1378] -> w1270
            tunnel: w1269 -> [w1377]
            tunnel: [w1377] -> w1268
            tunnel: w1267 -> [w1376]
            tunnel: [w1376] -> w1266
            tunnel: w1265 -> [w1371]
            tunnel: [w1370] -> w1264
            tunnel: [w1395] -> w1281
            tunnel: [w1394] -> w1280
            tunnel: [w1382] -> w1279
            tunnel: [w1383] -> w1278
            tunnel: [w1384] -> w1277
            tunnel: [w1379] -> w1276
            tunnel: w1274 -> [w1395]
            tunnel: w1272 -> [w1394]
            tunnel: w1270 -> [w1387]
            tunnel: w1268 -> [w1385]
            tunnel: w1266 -> [w1386]
            tunnel: w1264 -> [w1379]
            tunnel: [w1408] -> w1287
            tunnel: [w1410] -> w1286
            tunnel: [w1425] -> w1285
            tunnel: [w1424] -> w1284
            tunnel: [w1423] -> w1283
            tunnel: [w1397] -> w1282
            tunnel: w1281 -> [w1408]
            tunnel: w1280 -> [w1410]
            tunnel: w1279 -> [w1425]
            tunnel: w1278 -> [w1424]
            tunnel: w1277 -> [w1423]
            tunnel: w1276 -> [w1403]
            tunnel: [w1400] -> w1257
            tunnel: [w1453] -> w1256
            tunnel: [w1452] -> w1254
            tunnel: [w1435] -> w1252
            tunnel: [w1440] -> w1250
            tunnel: [w1444] -> w1248
            tunnel: [w1451] -> w1246
            tunnel: w1287 -> [w1453]
            tunnel: w1286 -> [w1452]
            tunnel: w1285 -> [w1446]
            tunnel: w1284 -> [w1447]
            tunnel: w1283 -> [w1445]
            tunnel: w1282 -> [w1451]
            tunnel: w1257 -> [w1436]
            tunnel: w1256 -> [w1463]
            tunnel: [w1463] -> w1255
            tunnel: w1254 -> [w1457]
            tunnel: [w1457] -> w1253
            tunnel: w1252 -> [w1462]
            tunnel: [w1462] -> w1251
            tunnel: w1250 -> [w1461]
            tunnel: [w1461] -> w1249
            tunnel: w1248 -> [w1460]
            tunnel: [w1460] -> w1247
            tunnel: w1246 -> [w1459]
            tunnel: [w1458] -> w1245
            tunnel: w1255 -> [w1472]
            tunnel: [w1472] -> w1293
            tunnel: w1253 -> [w1471]
            tunnel: [w1471] -> w1292
            tunnel: w1251 -> [w1470]
            tunnel: [w1470] -> w1291
            tunnel: w1249 -> [w1469]
            tunnel: [w1469] -> w1290
            tunnel: w1247 -> [w1468]
            tunnel: [w1468] -> w1289
            tunnel: w1245 -> [w1467]
            tunnel: [w1467] -> w1288
            tunnel: [w1479] -> w1331
            tunnel: [w1473] -> w1330
            tunnel: [w1477] -> w1329
            tunnel: [w1476] -> w1325
            tunnel: [w1475] -> w1307
            tunnel: [w1474] -> w1306
            tunnel: w1293 -> [w1474]
            tunnel: w1292 -> [w1475]
            tunnel: w1291 -> [w1481]
            tunnel: w1290 -> [w1482]
            tunnel: w1289 -> [w1480]
            tunnel: w1288 -> [w1477]
            tunnel: w1331 -> [w1503]
            tunnel: w1330 -> [w1505]
            tunnel: w1329 -> [w1506]
            tunnel: [w1501] -> w1328
            tunnel: [w1505] -> w1327
            tunnel: [w1504] -> w1326
            tunnel: w1325 -> [w1504]
            tunnel: [w1503] -> w1324
            tunnel: w1307 -> [w1497]
            tunnel: w1306 -> [w1498]
            tunnel: [w1498] -> w1304
            tunnel: [w1497] -> w1302
            tunnel: [w1491] -> w1295
            tunnel: w1328 -> [w1512]
            tunnel: w1327 -> [w1516]
            tunnel: w1326 -> [w1515]
            tunnel: w1324 -> [w1514]
            tunnel: [w1513] -> w1323
            tunnel: [w1512] -> w1322
            tunnel: [w1508] -> w1318
            tunnel: [w1511] -> w1316
            tunnel: [w1510] -> w1305
            tunnel: w1304 -> [w1510]
            tunnel: [w1509] -> w1303
            tunnel: w1302 -> [w1509]
            tunnel: w1323 -> [w1542]
            tunnel: w1322 -> [w1540]
            tunnel: [w1542] -> w1321
            tunnel: [w1534] -> w1320
            tunnel: [w1539] -> w1319
            tunnel: w1318 -> [w1539]
            tunnel: [w1538] -> w1317
            tunnel: w1316 -> [w1538]
            tunnel: w1305 -> [w1533]
            tunnel: w1303 -> [w1532]
            tunnel: [w1533] -> w1300
            tunnel: [w1532] -> w1298
            tunnel: [w1526] -> w1294
            tunnel: w1321 -> [w1549]
            tunnel: w1320 -> [w1543]
            tunnel: w1319 -> [w1550]
            tunnel: w1317 -> [w1548]
            tunnel: [w1543] -> w1315
            tunnel: [w1547] -> w1314
            tunnel: [w1546] -> w1301
            tunnel: w1300 -> [w1546]
            tunnel: [w1545] -> w1299
            tunnel: w1298 -> [w1545]
            tunnel: w1315 -> [w1567]
            tunnel: w1314 -> [w1568]
            tunnel: [w1568] -> w1312
            tunnel: [w1564] -> w1311
            tunnel: w1301 -> [w1563]
            tunnel: w1299 -> [w1560]
            tunnel: [w1560] -> w1296
            tunnel: [w1569] -> w1313
            tunnel: [w1577] -> w1310
            tunnel: w1312 -> [w1577]
            tunnel: w1311 -> [w1569]
            tunnel: [w1571] -> w1309
            tunnel: [w1570] -> w1297
            tunnel: w1296 -> [w1570]
            frame #0 {
              n325 = local write "Next Step"(FALSE ("Next Step")) -> ()
            }
            frame #1 {
              (unwired) FALSE ("Resize to Image Size? (Y)")
              # "configure projector"
              n326 = call "IMAQ FillImage"("Color Pixel Value"=u32 0, "error in (no error)"=w1350, "Image"=w1347) -> ("error out"=w1354:errorcluster, "Image Out"=w1346:T3)  [unwired: 7 in]
              n327 = call "prompt_user_for_projector_settings.vi"() -> ("blue exp_time_us out"=w1362:i32, "red exp_time_us out"=w1361:i32, "green exp_time_us out"=w1360:i32, "RedCurrent out"=w1359:u8, "RedBluePatternRepeat out"=w1342:i32, "GreenCurrent out"=w1358:u8, "BlueCurrent out"=w1357:u8, "projector params to save"=w1343:string[][])  [unwired: 4 in]
              n328 = while {
                stop <- w1364 stop-if-true
                n329 = local read "Next Step"() -> (w1364:bool)
                n330 = Wait (ms)(milliseconds to wait=u32 500) -> ()  [unwired: 1 out]
              }
              n331 = local write "Calibration Instructions"("Maker sure a plain agar plate is in place and IR is on. \nEnter in the correct projector configurations.") -> ()
              n332 = local write "Stimulus Image"(w1346) -> ()
              n333 = call "initialize_projector.vi"("BlueCurrent"=w1357, "RedBluePatternRepeat"=w1342, "GreenCurrent"=w1358, "RedCurrent"=w1359, "error in"=w1356, "blue exp_time_us"=w1362, "red exp_time_us"=w1361, "green exp_time_us"=w1360) -> ("error out"=w1355:errorcluster)  [unwired: 3 in]
              n334 = call "IMAQ Expand"("Y Duplication Step"=2, "error in (no error)"=w1354, "Image Dst"=w1351, "Image Src"=w1346) -> ("error out"=w1352:errorcluster, "Image Dst Out"=w1353:T3)  [unwired: 6 in]
              n335 = call "IMAQ WindDraw"("error in (no error)"=w1352, "Image"=w1353) -> ("error out"=w1349:errorcluster, "Image Out (duplicate)"=w1348:T3)  [unwired: 8 in]
            }
            frame #2 {
              # "get background"
              n336 = call "snap_single_image.vi"("error in (no error)"=w1371, "Session In"=w1369) -> ("error out"=w1374:errorcluster, "Image Out"=w1367:T3)  [unwired: 8 in]
              n337 = local write "Acquired Image"(w1367) -> ()
              n338 = local write "Next Step"(FALSE ("Next Step")) -> ()
              n339 = call "IMAQ Create"("Image Name"="background", "error in (no error)"=w1374) -> ("New Image"=w1372:T3, "error out"=w1373:errorcluster)  [unwired: 3 in]
              n340 = call "IMAQ Copy"("error in (no error)"=w1373, "Image Dst"=w1372, "Image Src"=w1367) -> ("error out"=w1370:errorcluster, "Image Dst Out"=w1368:T3)  [unwired: 3 in]
            }
            frame #3 {
              # "measure blue leackage"
              # "configure timing\n and current"
              n341 = global read "ParametersGlobal.vi" "Calibration Projector Dot Radius (projector pixel)"() -> (w1381:i32)
              n342 = global read "ParametersGlobal.vi" "Projector Calibration Points"() -> (w1380:cluster{"X":dbl, "Y":dbl}[])
              n343 = call "generate_spatial_calibration_pattern.vi"("Color Pixel Value"=u32 255, "error in (no error)"=w1387, "Dot Radius (Projector Pixels)"=w1381, "Points Array"=w1380, "StimulusImageIn"=w1385) -> ("error out"=w1393:errorcluster, "StimulusImageOut"=w1383:T3)  [unwired: 5 in]
              n344 = flat-sequence {
                tunnel: w1382 -> [_]
                frame #0 {
                  # "display update delay"
                  n345 = Wait (ms)(milliseconds to wait=200) -> ()  [unwired: 1 out]
                }
              }
              n346 = local write "Stimulus Image"(w1383) -> ()
              n347 = call "IMAQ Expand"("Y Duplication Step"=2, "error in (no error)"=w1393, "Image Dst"=w1386, "Image Src"=w1383) -> ("error out"=w1392:errorcluster, "Image Dst Out"=w1391:T3)  [unwired: 6 in]
              n348 = call "IMAQ WindDraw"("Resize to Image Size? (Y)"=FALSE, "error in (no error)"=w1392, "Image"=w1391) -> ("error out"=w1382:errorcluster, "Image Out (duplicate)"=w1384:T3)  [unwired: 7 in]
            }
            frame #4 {
              # "measure blue leackage"
              n349 = global read "ParametersGlobal.vi" "Tracking Binary Threshold Level"() -> (w1418:sgl)
              n350 = call "snap_single_image.vi"("error in (no error)"=w1403, "Session In"=w1410) -> ("error out"=w1407:errorcluster, "Image Out"=w1402:T3)  [unwired: 8 in]
              n351 = local write "Acquired Image"(w1402) -> ()
              n352 = call "IMAQ Create"("Image Name"="processedagar", "error in (no error)"=w1407) -> ("New Image"=w1405:T3, "error out"=w1406:errorcluster)  [unwired: 3 in]
              n353 = local write "Calibration Instructions"("Confirm blue leakage is not outside of the temporal calibration zone.") -> ()
              n354 = call "IMAQ Copy"("error in (no error)"=w1406, "Image Dst"=w1405, "Image Src"=w1402) -> ("error out"=w1414:errorcluster, "Image Dst Out"=w1415:T3)  [unwired: 3 in]
              n355 = Bundle By Name(cluster=cluster{"Lower value":sgl, "Upper value":sgl} {"Lower value"=0.0, "Upper value"=255.0} ("Range"), "Lower value"=w1418) -> (w1416:cluster{"Lower value":sgl, "Upper value":sgl})
              n356 = call "IMAQ Subtract"("Image Src A"=w1415, "Image Dst"=w1415, "Image Src B"=w1408, "error in (no error)"=w1414) -> ("Image Dst Out"=w1419:T3, "error out"=w1417:errorcluster)  [unwired: 3 in]
              n357 = call "IMAQ Threshold"("Replace Value"=sgl 255.0, "Keep/Replace Value (Replace)"=TRUE, "error in (no error)"=w1417, "Range"=w1416, "Image Src"=w1419) -> ("error out"=w1420:errorcluster, "Image Dst Out"=w1422:T3)  [unwired: 5 in]
              n358 = global read "ParametersGlobal.vi" "Projector Camera Calibration Image"() -> (w1399:T3)
              n359 = call "white_out_TC_zone.vi"("error in (no error)"=w1420, "Refnum in"=w1422) -> ("error out"=w1398:errorcluster, "Refnum out"=w1421:T3)  [unwired: 8 in]
              n360 = global read "ParametersGlobal.vi" "TC Number of Time Bits Encoded"() -> (w1401:i32)
              n361 = local write "Processed Image"(w1421) -> ()
              n362 = while {
                stop <- w1430 stop-if-true
                n363 = local read "Next Step"() -> (w1430:bool)
                n364 = Wait (ms)(milliseconds to wait=u32 500) -> ()  [unwired: 1 out]
              }
              n365 = for {
                N: w1401 -> [_]
                tunnel: [w1427] -> w1400 mode=indexing
                i -> [w1429]
                n366 = Quotient & Remainder(x=w1429, y=2) -> (x-y*floor(x/y)=w1428:i32)  [unwired: 1 out]
                n367 = Equal To 0?(x=w1428) -> (x = 0?=w1427:bool)
              }
              n368 = call "update_temporal_calibration_locations.vi"("error in (no error)"=w1398, "Projector to Camera Calibration in"=w1399) -> ("error out"=w1397:errorcluster)  [unwired: 9 in]
            }
            frame #5 {
              # "preview temporal calibration"
              n369 = call "IMAQ FillImage"("Color Pixel Value"=u32 0, "error in (no error)"=w1446, "Image"=w1447) -> ("error out"=w1443:errorcluster, "Image Out"=w1441:T3)  [unwired: 7 in]
              n370 = global read "ParametersGlobal.vi" "TC Zero XY values (Projector Pixels)"() -> (w1438:i32[][])
              n371 = global read "ParametersGlobal.vi" "TC One XY values (Projector Pixels)"() -> (w1437:i32[][])
              n372 = global read "ParametersGlobal.vi" "TC Dot Radius (Projector Pixels)"() -> (w1439:i32)
              n373 = local write "Next Step"(FALSE ("Next Step")) -> ()
              n374 = call "draw_temporal_calibration.vi"("TC One XY values (Projector Pixels)"=w1437, "TC Zero XY values (Projector Pixels)"=w1438, "error in (no error)"=w1443, "Buffer  Bits To Be Encoded"=w1436, "TC Dot Radius (Projector Pixels)"=w1439, "Image in"=w1441) -> ("error out"=w1442:errorcluster, "Image Out"=w1440:T3)  [unwired: 3 in]
              n375 = local write "Stimulus Image"(w1440) -> ()
              n376 = flat-sequence {
                tunnel: w1435 -> [_]
                frame #0 {
                  # "display update delay"
                  n377 = Wait (ms)(milliseconds to wait=200) -> ()  [unwired: 1 out]
                }
              }
              n378 = call "IMAQ Expand"("Y Duplication Step"=2, "error in (no error)"=w1442, "Image Dst"=w1445, "Image Src"=w1440) -> ("error out"=w1449:errorcluster, "Image Dst Out"=w1450:T3)  [unwired: 6 in]
              n379 = call "IMAQ WindDraw"("Resize to Image Size? (Y)"=FALSE, "error in (no error)"=w1449, "Image"=w1450) -> ("error out"=w1435:errorcluster, "Image Out (duplicate)"=w1444:T3)  [unwired: 7 in]
            }
            frame #6 {
              # "preview temporal calibration"
              n380 = call "snap_single_image.vi"("error in (no error)"=w1459, "Session In"=w1457) -> ("error out"=w1458:errorcluster, "Image Out"=w1456:T3)  [unwired: 8 in]
              n381 = local write "Acquired Image"(w1456) -> ()
              n382 = local write "Calibration Instructions"("Confirm temporal calibration has good signal.") -> ()
              n383 = while {
                stop <- w1464 stop-if-true
                n384 = local read "Next Step"() -> (w1464:bool)
                n385 = Wait (ms)(milliseconds to wait=u32 500) -> ()  [unwired: 1 out]
              }
            }
            frame #7 {
              n386 = local write "Next Step"(FALSE ("Next Step")) -> ()
            }
            frame #8 {
              n387 = while {
                stop <- w1489 stop-if-true
                n388 = local read "Next Step"() -> (w1489:bool)
                n389 = Wait (ms)(milliseconds to wait=u32 500) -> ()  [unwired: 1 out]
              }
              n390 = local write "Calibration Instructions"("Load power meter plate.\nSet the wavelength to 635nm.\nTurn off IR." ("Calibration Instructions")) -> ()
              n391 = call "IMAQ FillImage"("Color Pixel Value"=u32 16711680, "error in (no error)"=w1481, "Image"=w1482) -> ("error out"=w1483:errorcluster, "Image Out"=w1473:T3)  [unwired: 7 in]
              n392 = local write "Stimulus Image"(w1473) -> ()
              n393 = call "IMAQ Expand"("Y Duplication Step"=2, "error in (no error)"=w1483, "Image Dst"=w1480, "Image Src"=w1473) -> ("error out"=w1485:errorcluster, "Image Dst Out"=w1484:T3)  [unwired: 6 in]
              n394 = call "IMAQ WindDraw"("Resize to Image Size? (Y)"=FALSE, "error in (no error)"=w1485, "Image"=w1484) -> ("error out"=w1479:errorcluster, "Image Out (duplicate)"=w1476:T3)  [unwired: 7 in]
            }
            frame #9 {
              n395 = local read "Power Meter Probe Area (mm^2)"() -> (w1496:dbl)
              n396 = local write "Next Step"(FALSE ("Next Step")) -> ()
              n397 = call "snap_single_image.vi"("error in (no error)"=w1506, "Session In"=w1497) -> ("error out"=w1502:errorcluster, "Image Out"=w1499:T3)  [unwired: 8 in]
              n398 = call "IMAQ Copy"("error in (no error)"=w1502, "Image Dst"=w1498, "Image Src"=w1499) -> ("error out"=w1501:errorcluster, "Image Dst Out"=w1500:T3)  [unwired: 3 in]
              n399 = call "prompt_user_for_number_input.vi"() -> ("Power Reading out"=w1493:dbl)  [unwired: 6 in]
              n400 = local write "Acquired Image"(w1500) -> ()
              n401 = Divide(x=w1493, y=w1496) -> (x/y=w1494:dbl)
              n402 = Number To Fractional String(number=w1494) -> (F-format string=w1495:string)  [unwired: 3 in]
              n403 = Build Array("avgPowerRed", w1495) -> (w1491:string[])
            }
            frame #10 {
              n404 = local write "Calibration Instructions"("Set the wavelength to 540nm" ("Calibration Instructions")) -> ()
              n405 = while {
                stop <- w1525 stop-if-true
                n406 = local read "Next Step"() -> (w1525:bool)
                n407 = Wait (ms)(milliseconds to wait=u32 500) -> ()  [unwired: 1 out]
              }
              n408 = call "IMAQ FillImage"("Color Pixel Value"=u32 65280, "error in (no error)"=w1514, "Image"=w1516) -> ("error out"=w1518:errorcluster, "Image Out"=w1508:T3)  [unwired: 7 in]
              n409 = call "IMAQ Expand"("Y Duplication Step"=2, "error in (no error)"=w1518, "Image Dst"=w1515, "Image Src"=w1508) -> ("error out"=w1520:errorcluster, "Image Dst Out"=w1519:T3)  [unwired: 6 in]
              n410 = local write "Stimulus Image"(w1508) -> ()
              n411 = call "IMAQ WindDraw"("Resize to Image Size? (Y)"=FALSE, "error in (no error)"=w1520, "Image"=w1519) -> ("error out"=w1513:errorcluster, "Image Out (duplicate)"=w1511:T3)  [unwired: 7 in]
            }
            frame #11 {
              n412 = local read "Power Meter Probe Area (mm^2)"() -> (w1531:dbl)
              n413 = call "snap_single_image.vi"("error in (no error)"=w1540, "Session In"=w1532) -> ("error out"=w1537:errorcluster, "Image Out"=w1536:T3)  [unwired: 8 in]
              n414 = local write "Next Step"(FALSE ("Next Step")) -> ()
              n415 = call "IMAQ Copy"("error in (no error)"=w1537, "Image Dst"=w1533, "Image Src"=w1536) -> ("error out"=w1534:errorcluster, "Image Dst Out"=w1535:T3)  [unwired: 3 in]
              n416 = call "prompt_user_for_number_input.vi"() -> ("Power Reading out"=w1530:dbl)  [unwired: 6 in]
              n417 = local write "Acquired Image"(w1535) -> ()
              n418 = Divide(x=w1530, y=w1531) -> (x/y=w1528:dbl)
              n419 = Number To Fractional String(number=w1528) -> (F-format string=w1529:string)  [unwired: 3 in]
              n420 = Build Array("avgPowerGreen", w1529) -> (w1526:string[])
            }
            frame #12 {
              n421 = while {
                stop <- w1559 stop-if-true
                n422 = local read "Next Step"() -> (w1559:bool)
                n423 = Wait (ms)(milliseconds to wait=u32 500) -> ()  [unwired: 1 out]
              }
              n424 = local write "Calibration Instructions"("Set the wavelength to 455nm" ("Calibration Instructions")) -> ()
              n425 = call "IMAQ FillImage"("Color Pixel Value"=u32 255, "error in (no error)"=w1549, "Image"=w1550) -> ("error out"=w1552:errorcluster, "Image Out"=w1544:T3)  [unwired: 7 in]
              n426 = call "IMAQ Expand"("Y Duplication Step"=2, "error in (no error)"=w1552, "Image Dst"=w1548, "Image Src"=w1544) -> ("error out"=w1554:errorcluster, "Image Dst Out"=w1553:T3)  [unwired: 6 in]
              n427 = local write "Stimulus Image"(w1544) -> ()
              n428 = call "IMAQ WindDraw"("Resize to Image Size? (Y)"=FALSE, "error in (no error)"=w1554, "Image"=w1553) -> ("error out"=w1547:errorcluster)  [unwired: 7 in, 1 out]
            }
            frame #13 {
              n429 = call "snap_single_image.vi"("error in (no error)"=w1567, "Session In"=w1560) -> ("error out"=w1565:errorcluster, "Image Out"=w1562:T3)  [unwired: 8 in]
              n430 = call "IMAQ Copy"("error in (no error)"=w1565, "Image Dst"=w1563, "Image Src"=w1562) -> ("error out"=w1564:errorcluster, "Image Dst Out"=w1561:T3)  [unwired: 3 in]
              n431 = local write "Next Step"(FALSE ("Next Step")) -> ()
              n432 = local write "Acquired Image"(w1561) -> ()
            }
            frame #14 {
              n433 = local read "Power Meter Probe Area (mm^2)"() -> (w1572:dbl)
              n434 = call "prompt_user_for_number_input.vi"() -> ("Power Reading out"=w1573:dbl)  [unwired: 6 in]
              n435 = Divide(x=w1573, y=w1572) -> (x/y=w1576:dbl)
              n436 = Number To Fractional String(number=w1576) -> (F-format string=w1574:string)  [unwired: 3 in]
              n437 = Build Array("avgPowerBlue", w1574) -> (w1571:string[])
            }
          }
        }
        frame True {
        }
      }
      n438 = Build Array (concatenate)(w1221, w1215) -> (w1220:string[][])
      n439 = Build Array (concatenate)(w1220, w1227) -> (w1231:string[][])
      n440 = Build Array (concatenate)(w1231, w1226) -> (w1230:string[][])
      n441 = Build Array (concatenate)(w1230, w1229) -> (w1228:string[][])
      n442 = call <vilib>:"IMAQdx Stop Acquisition.vi"("error in"=w1233, "Session In"=w1234) -> ("error out"=w1241:errorcluster, "Session Out"=w1242:T8)  [unwired: 8 in]
      n443 = call <vilib>:"IMAQdx Unconfigure Acquisition.vi"("error in"=w1241, "Session In"=w1242) -> ("error out"=w1244:errorcluster, "Session Out"=w1243:T8)  [unwired: 8 in]
      n444 = flat-sequence {
        tunnel: w1235 -> [_]
        frame #0 {
          n445 = local write "Calibration Instructions"("Calibration Complete" ("Calibration Instructions")) -> ()
        }
      }
      n446 = call "IMAQ WindClose"("error in (no error)"=w1232) -> ("error out"=w1236:errorcluster)  [unwired: 5 in]
      n447 = call <vilib>:"IMAQdx Close Camera.vi"("error in"=w1244, "Session In"=w1243) -> ("error out"=w1240:errorcluster)  [unwired: 9 in]
      n448 = Merge Errors(w1240, w1236) -> (w1239:errorcluster)
      n449 = case shown="No Error" w1239 {
        selector: w1239 -> [w1582 w1586]
        tunnel: [w1585 w1586] -> w1238
        tunnel: w1228 -> [w1584 _]
        tunnel: w1237 -> [w1583 _]
        frame No Error {
          n450 = call "write_parameters_csv_from_calibration.vi"("error in (no error)"=w1582, "parameter, value pairs"=w1584, "Computer Name"=w1583) -> ("error out"=w1585:errorcluster)  [unwired: 8 in]
        }
        frame Error {
        }
      }
      n451 = call <vilib>:"General Error Handler.vi"("error in (no error)"=w1238) -> ("error out"=w1235:errorcluster)  [unwired: 10 in, 4 out]
    }
  }
  "error out" <- w15
  "Parameters Written" <- w14
